vi "ADIS16470 Loop.vi"(8 "error in":errorcluster) -> ()   [LabVIEW 2019]
uses:
  Typedef/ADIS16470 Device Reference.ctl
  Typedef/ADIS16470 Hardware Configuration.ctl
  <vilib>/Rock Robotics/WPI/SPI/WPI_SPIMode.ctl
  <vilib>/Rock Robotics/SystemInterfaces/DIO/FPGA_DIOChannel.ctl
  <vilib>/Rock Robotics/SystemInterfaces/spilib/spi_bus.ctl
  Typedef/ADIS16470 Status.ctl
  Typedef/ADIS16470 Data.ctl
  Typedef/ADIS16470 Process.ctl
  Typedef/ADIS16470 Command Type.ctl
  <vilib>/Rock Robotics/SystemInterfaces/CounterEncoderSourceConvertion/FPGA_CounterEncoderSourceConvertionLVSourceType.ctl
  <vilib>/Rock Robotics/SystemInterfaces/DIO/FPGA_DIODigitalSourceChannel.ctl
  <vilib>/Rock Robotics/SystemInterfaces/AnalogTrigger/FPGA_AnalogTriggerIndex.ctl
  <vilib>/Rock Robotics/SystemInterfaces/AnalogTrigger/FPGA_AnalogTriggerOutType.ctl
  Typedef/ADIS16470 Calibration Time.ctl
  Typedef/ADIS16470 Loop Data.ctl
  <vilib>/Rock Robotics/WPI/SPI/WPI_SPIDevRef.ctl
  Typedef/ADIS16470 Register.ctl
  Typedef/ADIS16470 Loop State.ctl
  Typedef/ADIS16470 Register Read Info.ctl
  <vilib>/Rock Robotics/WPI/Counter/WPI_CounterDigitalInputToDigitalSource.vi
  <vilib>/Rock Robotics/WPI/ThirdParty/JAS_Junk/TrajLib/Trajectory_Library.lvlib
panel:
  in  "Use Register Read Mode":bool
  in  "Calibration Time":T1
  in  "element":T2
  out "Offset Bias":i16[](array[numeric])
  in  "ADIS16470DevRef":T3={"DevStatus"={"status"=FALSE, "code"=0, "source"=""}, "Hardware Config"={"SPI Clock Rate (Hz)"=1000000.0, "IMU SPI Mode (3)"=enum."Mode 3 (Clk Idle High,Sample on Trailing)", "IMU Reset Pin"=enum."SPI Port CS2", "IMU SPI Bus"=enum."SPI On-Board, CS0", "IMU Data Ready Pin"=enum."SPI Port CS1", "Stall Config"={"Pow2BytesPerRead"=255, "StallTicks"=640, "CsToSclkTicks"=5}}, "Calibration Complete"=refnum, "Status FIFO"=refnum, "Last Value Reference"=refnum, "Sychronous Process VI"=refnum, "Cmd FIFO"=refnum, "Source"={"DevStatus"={"status"=FALSE, "code"=0, "source"=""}, "AnalogTriggerMode?"=FALSE, "DigitalMode"={"DIO Channel"=enum."Disabled"}, "AnalogTriggerMode"={"AnalogTriggerIndex"=enum."Trig 0", "OutputType"=enum."InWindow"}}, "Data FIFO"=refnum, "Calibration Time"=enum."1s"}
  in  "Main Name":string
  # "XG_BIAS_LOW"
  # "XG_BIAS_HIGH"
  # "YG_BIAS_LOW"
  # "YG_BIAS_HIGH"
  # "ZG_BIAS_LOW"
  # "ZG_BIAS_HIGH"
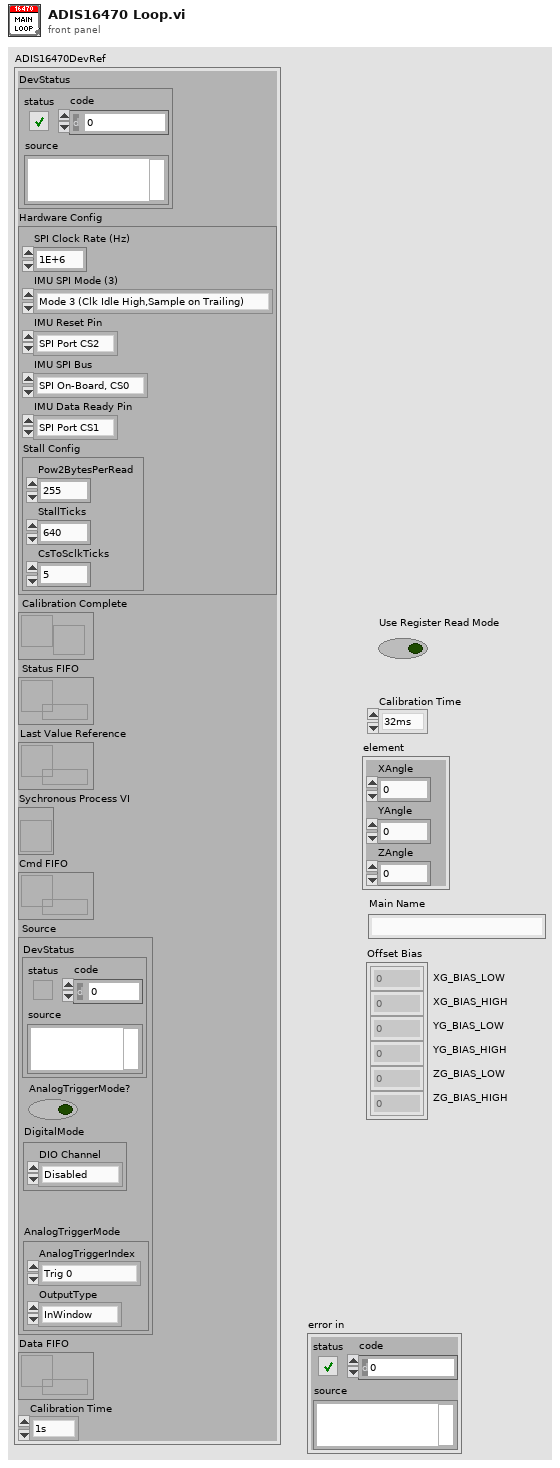
[diagram p1: front panel]
types:
  T1 = typedef "ADIS16470 Calibration Time.ctl" = enum16{"32ms", "64ms", "128ms", "256ms", "512ms", "1s", "2s", "4s", "8s", "16s", "32s", "64s"}
  T2 = typedef "ADIS16470 Data.ctl" = cluster{"XAngle":dbl, "YAngle":dbl, "ZAngle":dbl}
  T3 = typedef "ADIS16470 Device Reference.ctl" = cluster{"DevStatus":errorcluster, "Hardware Config":T4, "Calibration Complete":refnum<notifier>, "Status FIFO":refnum<k33>, "Last Value Reference":refnum<data-value>, "Sychronous Process VI":T8, "Cmd FIFO":refnum<k33>, "Source":T9, "Data FIFO":refnum<k33>, "Calibration Time":T1}
  T4 = typedef "ADIS16470 Hardware Configuration.ctl" = cluster{"SPI Clock Rate (Hz)":dbl, "IMU SPI Mode (3)":T5, "IMU Reset Pin":T6, "IMU SPI Bus":T7, "IMU Data Ready Pin":T6, "Stall Config":cluster{"Pow2BytesPerRead":u8, "StallTicks":u16, "CsToSclkTicks":u8}}
  T5 = typedef "WPI_SPIMode.ctl" = enum16{"Mode 0 (Clk Idle Low,Sample on Leading)", "Mode 1 (Clk Idle Low,Sample on Trailing)", "Mode 2 (Clk Idle High,Sample on Leading)", "Mode 3 (Clk Idle High,Sample on Trailing)"}
  T6 = typedef "FPGA_DIOChannel.ctl" = enum8{"DIO 0", "DIO 1", "DIO 2", "DIO 3", "DIO 4", "DIO 5", "DIO 6", "DIO 7", "DIO 8", "DIO 9", "DIO MXP 0", "DIO MXP 1", "DIO MXP 2", "DIO MXP 3", "DIO MXP 4", "DIO MXP 5", "DIO MXP 6", "DIO MXP 7", "DIO MXP 8", "DIO MXP 9", "DIO MXP 10", "DIO MXP 11", "DIO MXP 12", "DIO MXP 13", "DIO MXP 14", "DIO MXP 15", "SPI Port CS1", "SPI Port CS2", "SPI Port CS3", "SPI Port MISO", "SPI Port MOSI", "Invalid"}
  T7 = typedef "spi_bus.ctl" = enum16{"SPI On-Board, CS0", "SPI On-Board, CS1", "SPI On-Board, CS2", "SPI On-Board, CS3", "SPI MXP", "Invalid"}
  T8 = typedef "ADIS16470 Process.ctl" = refnum<vi>
  T9 = typedef "FPGA_CounterEncoderSourceConvertionLVSourceType.ctl" = cluster{"DevStatus":errorcluster, "AnalogTriggerMode?":bool, "DigitalMode":cluster{"DIO Channel":T10}, "AnalogTriggerMode":cluster{"AnalogTriggerIndex":T11, "OutputType":T12}}
  T10 = typedef "FPGA_DIODigitalSourceChannel.ctl" = enum8{"DIO 0", "DIO 1", "DIO 2", "DIO 3", "DIO 4", "DIO 5", "DIO 6", "DIO 7", "DIO 8", "DIO 9", "DIO MXP 0", "DIO MXP 1", "DIO MXP 2", "DIO MXP 3", "DIO MXP 4", "DIO MXP 5", "DIO MXP 6", "DIO MXP 7", "DIO MXP 8", "DIO MXP 9", "DIO MXP 10", "DIO MXP 11", "DIO MXP 12", "DIO MXP 13", "DIO MXP 14", "DIO MXP 15", "SPI Port CS1", "SPI Port CS2", "SPI Port CS3", "SPI Port MISO", "SPI Port MOSI", "Disabled"}
  T11 = typedef "FPGA_AnalogTriggerIndex.ctl" = enum8{"Trig 0", "Trig 1", "Trig 2", "Trig 3", "Trig 4", "Trig 5", "Trig 6", "Trig 7", "Invalid"}
  T12 = typedef "FPGA_AnalogTriggerOutType.ctl" = enum16{"InWindow", "TriggerState", "Rising", "Falling"}
  T13 = typedef "ADIS16470 Register Read Info.ctl" = cluster{"Reg":T14, "ByteInx":i32}[]
  T14 = typedef "ADIS16470 Register.ctl" = u8
  T15 = typedef "ADIS16470 Loop State.ctl" = enum16{"Default", "Error", "**Initialization**", "Reset", "Register DR Source", "Start SPI", "Write Config", "** Calibration **", "Calibrate", "Write Run Config", "Init Auto SPI", "** Operation **", "Run", "Process", "Run Cmds", "** Register Read Operation **", "Run Alt", "Run Cmds Alt"}
  T16 = typedef "ADIS16470 Loop Data.ctl" = cluster{"SPIDevRef":T17, "Data Counter":u16, "Reset":bool, "Digital Source":T9, "Bytes Per Sample":u32, "Data":dbl[], "ADIS16470DevRef":T3, "TimeStampPrev":u32, "Sensor to Robot Rotation":dbl[][], "Data Packet":T14[], "AutoSPI Active?":bool}
  T17 = typedef "WPI_SPIDevRef.ctl" = cluster{"DevStatus":errorcluster, "Handle":i32, "SPI Bus":T7}
  T18 = enum32{"Bad", "Idle", "Run top level", "Running"}
  T19 = typedef "ADIS16470 Status.ctl" = cluster{"Calibrated?":bool, "IMU Detected?":bool}
  T20 = typedef "ADIS16470 Command Type.ctl" = cluster{"Command":enum16{"None", "Reset", "Set Calibration Period", "Recalibrate", "Recal Complete", "Exit Auto SPI", "Start Auto SPI"}, "Data":u32}
  T21 = typedef "WPI_DigitalOutputDevRef.ctl" = cluster{"DIO Channel":T6, "DevStatus":errorcluster}
  T22 = typedef "WPI_DigitalInputDevRef.ctl" = cluster{"DevStatus":errorcluster, "DIO Channel":T6}
  T23 = cluster{"Pow2BytesPerRead":u8, "StallTicks":u16, "CsToSclkTicks":u8}
  T24 = enum16{"None", "Reset", "Set Calibration Period", "Recalibrate", "Recal Complete", "Exit Auto SPI", "Start Auto SPI"}
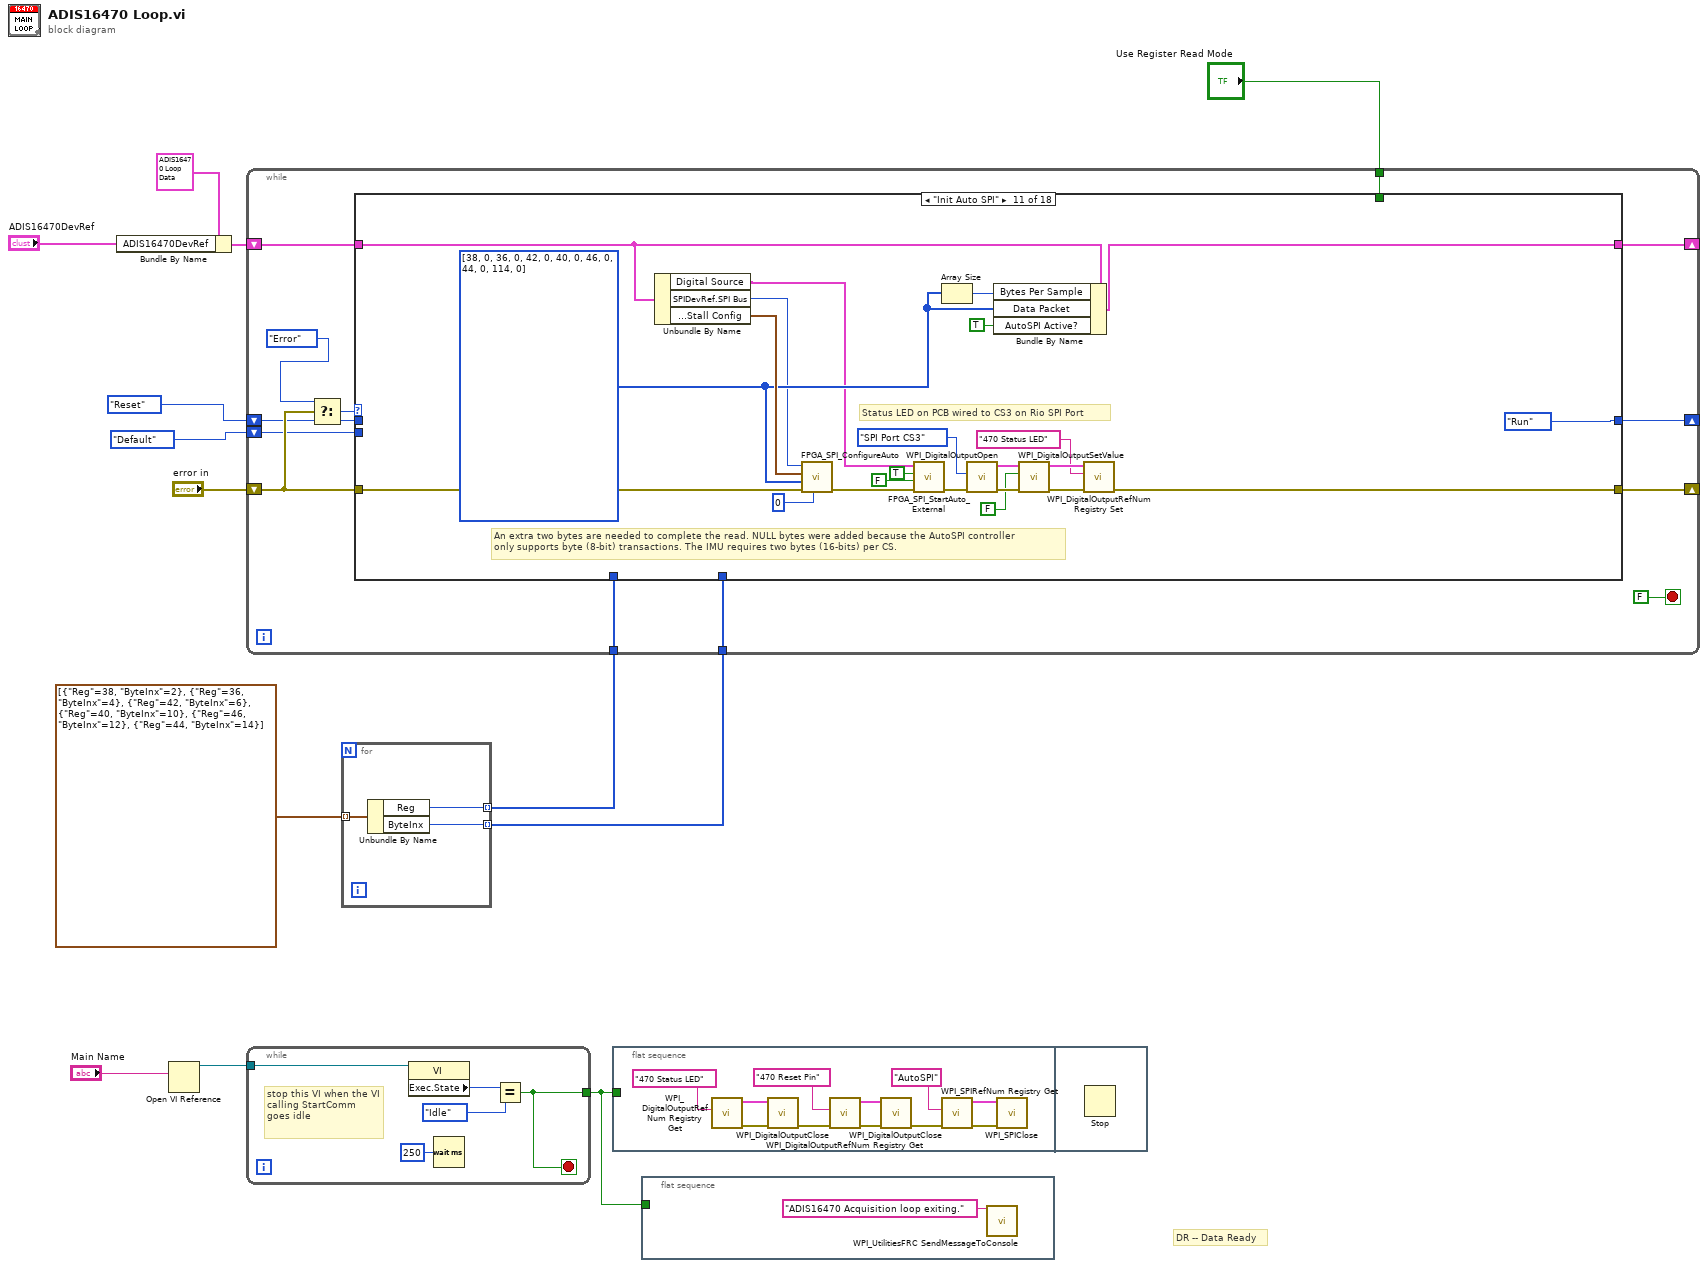
[diagram p0: block diagram]
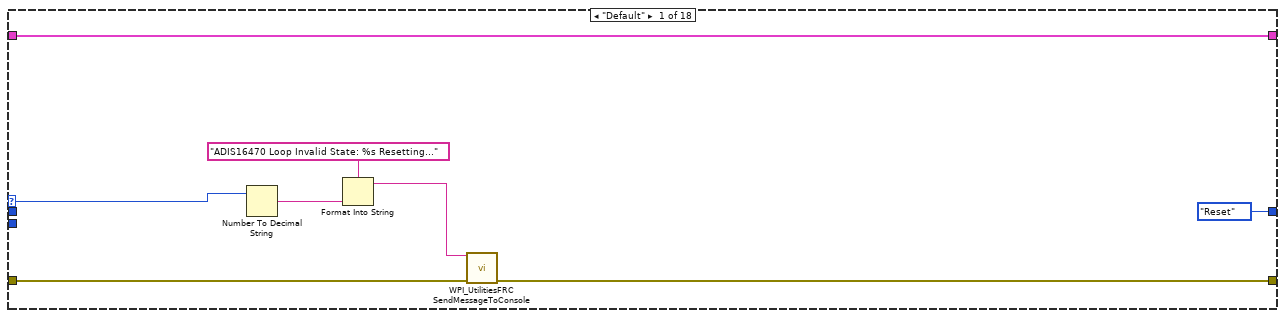
[diagram p2: hidden frame]
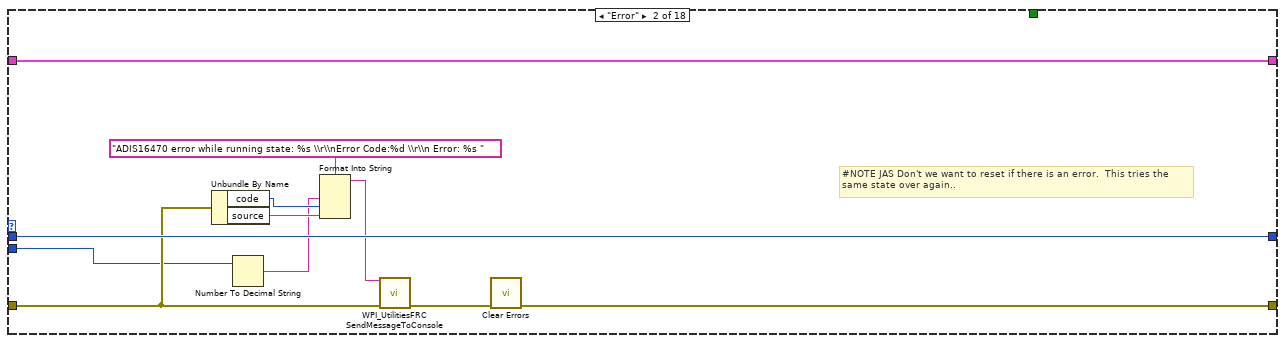
[diagram p3: hidden frame]
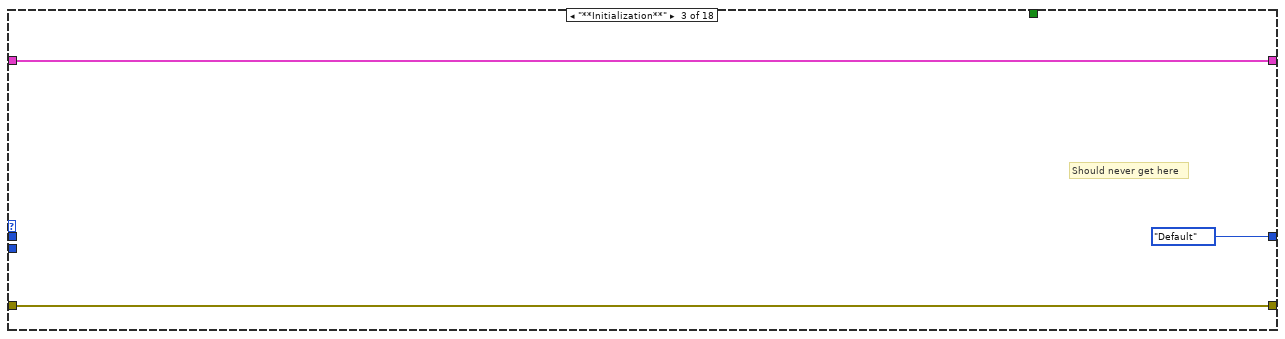
[diagram p4: hidden frame]
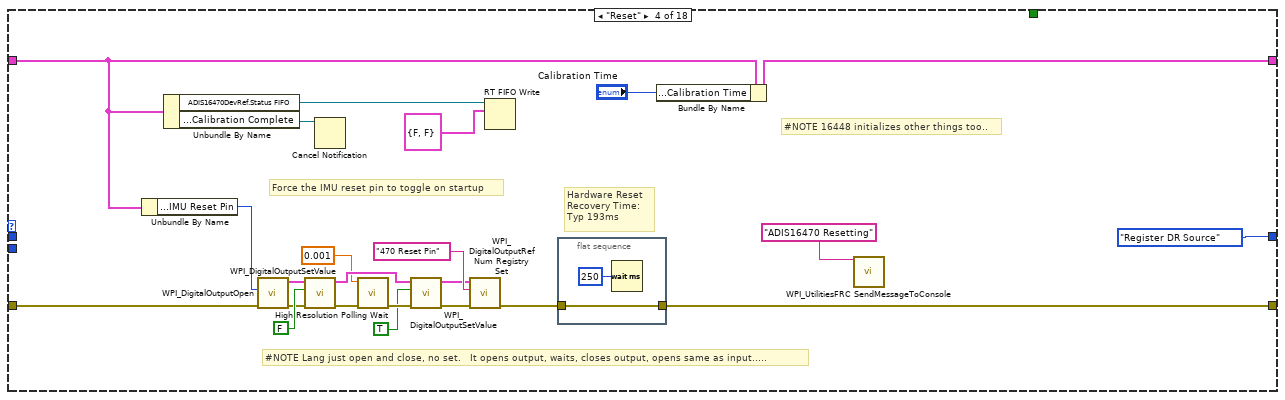
[diagram p5: hidden frame]
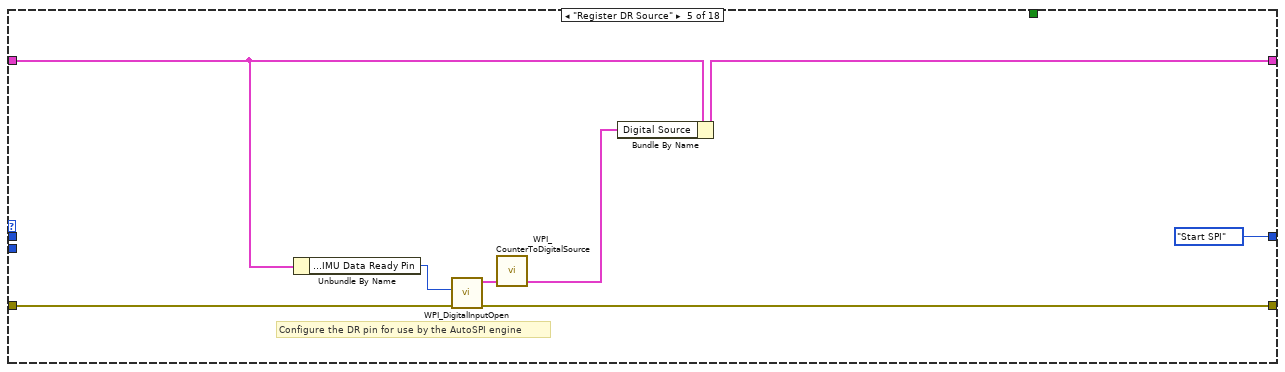
[diagram p6: hidden frame]
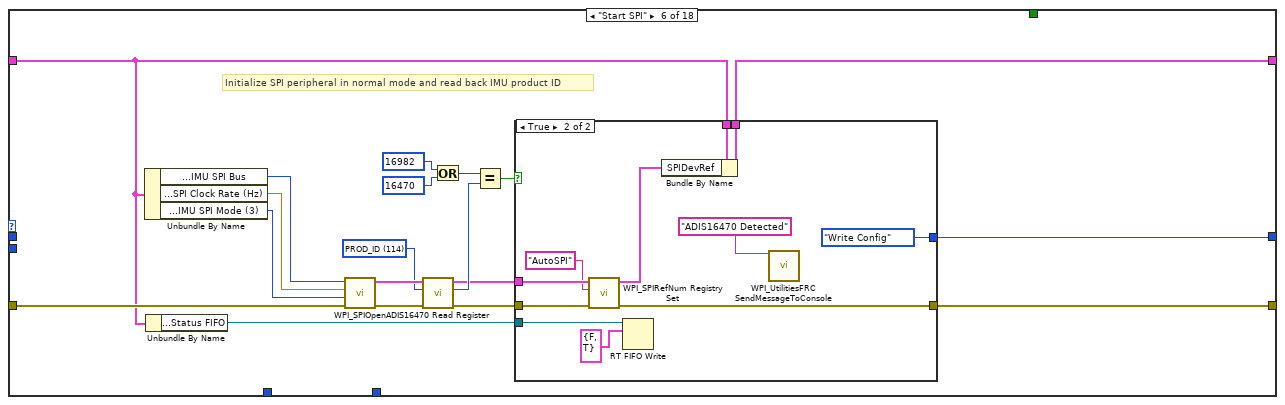
[diagram p7: hidden frame]
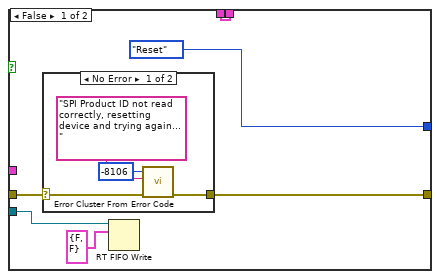
[diagram p8: hidden frame]
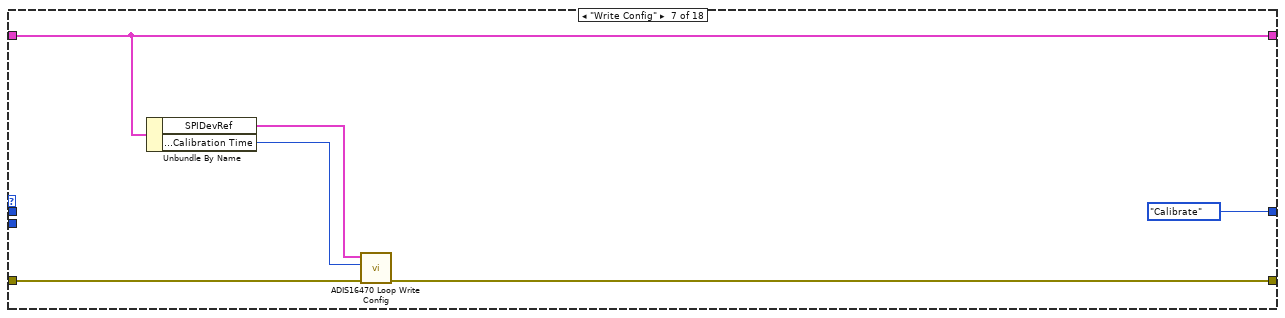
[diagram p10: hidden frame]
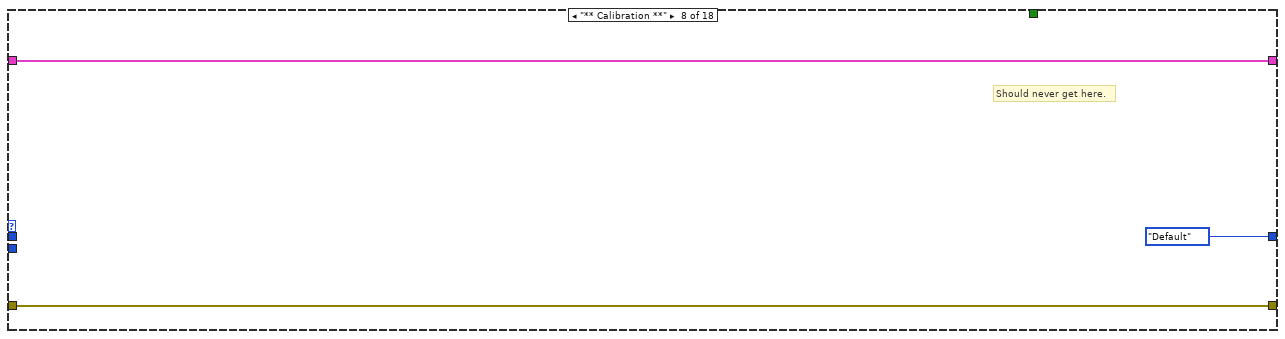
[diagram p11: hidden frame]
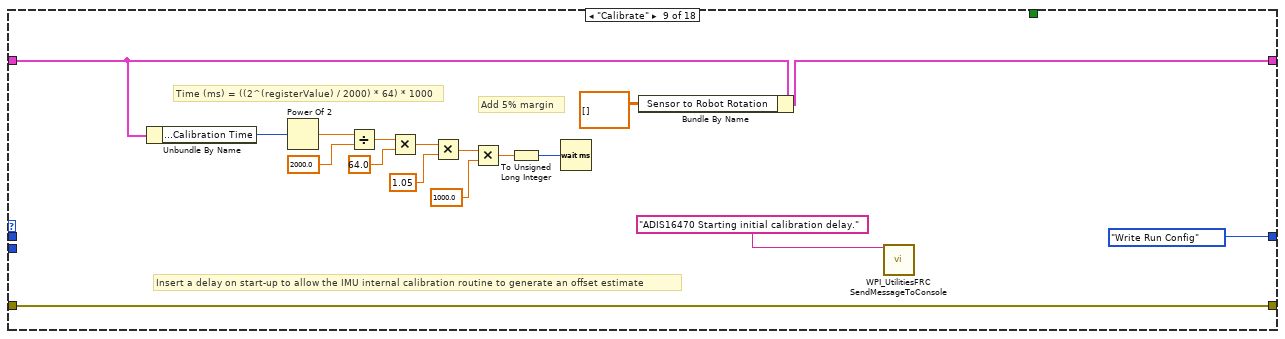
[diagram p12: hidden frame]
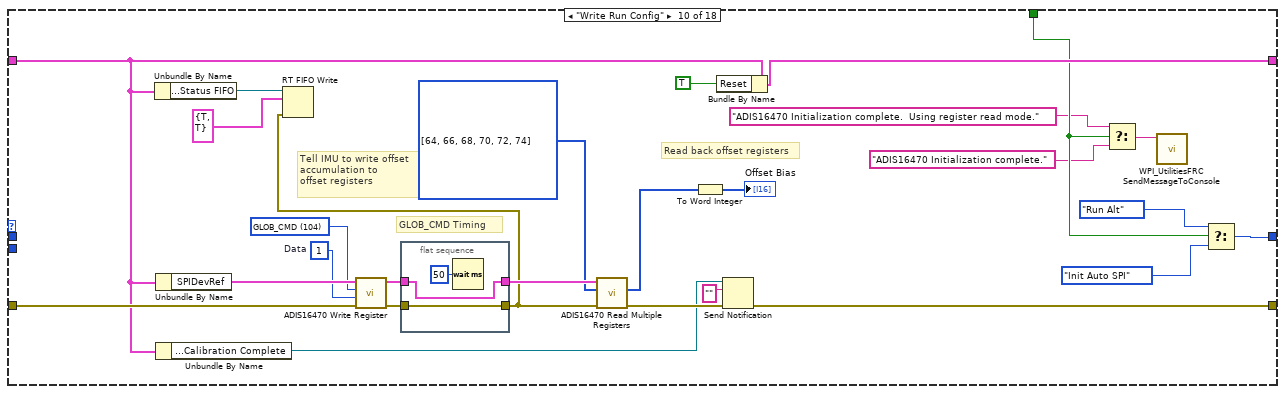
[diagram p13: hidden frame]
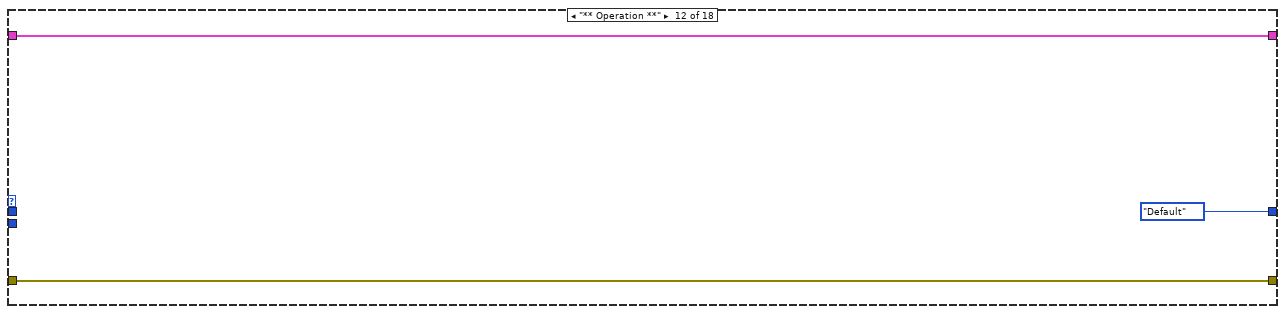
[diagram p14: hidden frame]
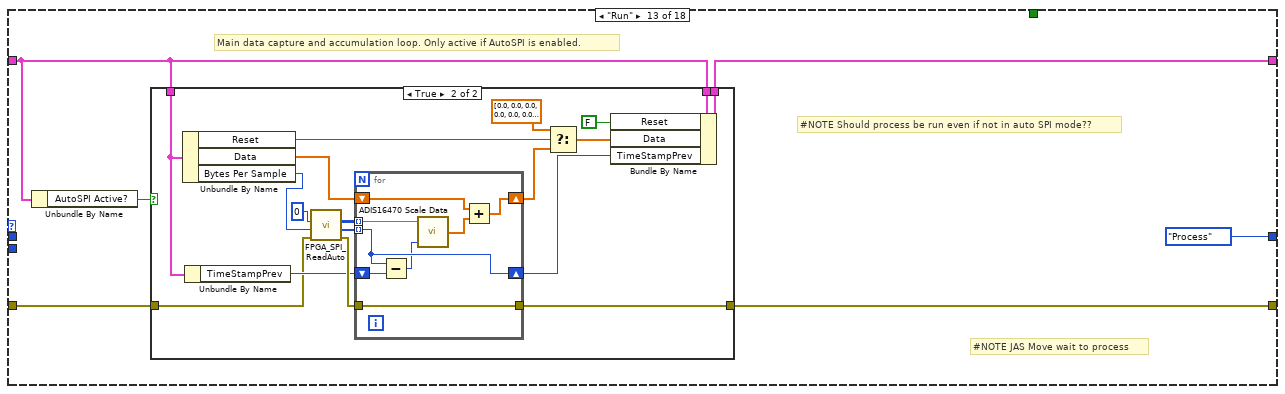
[diagram p15: hidden frame]
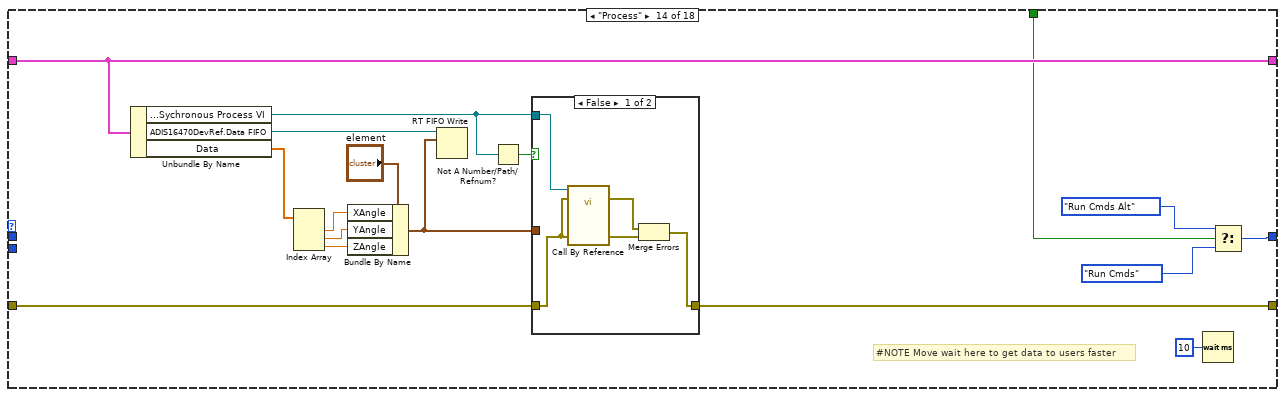
[diagram p17: hidden frame]
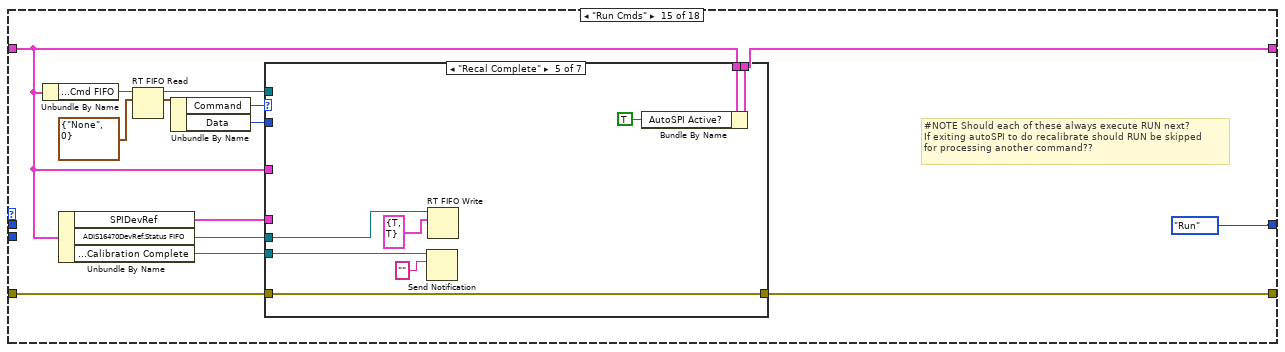
[diagram p19: hidden frame]
diagram:
  # "DR -- Data Ready"
  n1 = Bundle By Name(cluster=T16 {"SPIDevRef"={"DevStatus"={"status"=FALSE, "code"=0, "source"=""}, "Handle"=0, "SPI Bus"=enum."SPI On-Board, CS0"}, "Data Counter"=0, "Reset"=FALSE, "Digital Source"={"DevStatus"={"status"=FALSE, "code"=0, "source"=""}, "AnalogTriggerMode?"=FALSE, "DigitalMode"={"DIO Channel"=enum."DIO 1"}, "AnalogTriggerMode"={"AnalogTriggerIndex"=enum."Trig 0", "OutputType"=enum."InWindow"}}, "Bytes Per Sample"=0, "Data"=[0.0, 0.0, 0.0, 0.0, 0.0, 0.0, 0.0, 0.0], "ADIS16470DevRef"={"DevStatus"={"status"=FALSE, "code"=0, "source"=""}, "Hardware Config"={"SPI Clock Rate (Hz)"=1000000.0, "IMU SPI Mode (3)"=enum."Mode 3 (Clk Idle High,Sample on Trailing)", "IMU Reset Pin"=enum."SPI Port CS2", "IMU SPI Bus"=enum."SPI On-Board, CS0", "IMU Data Ready Pin"=enum."SPI Port CS1", "Stall Config"={"Pow2BytesPerRead"=255, "StallTicks"=640, "CsToSclkTicks"=5}}, "Calibration Complete"=refnum, "Status FIFO"=refnum, "Last Value Reference"=refnum, "Sychronous Process VI"=refnum, "Cmd FIFO"=refnum, "Source"={"DevStatus"={"status"=FALSE, "code"=0, "source"=""}, "AnalogTriggerMode?"=FALSE, "DigitalMode"={"DIO Channel"=enum."Disabled"}, "AnalogTriggerMode"={"AnalogTriggerIndex"=enum."Trig 0", "OutputType"=enum."InWindow"}}, "Data FIFO"=refnum, "Calibration Time"=enum."1s"}, "TimeStampPrev"=0, "Sensor to Robot Rotation"=[], "Data Packet"=[38, 0, 36, 0, 42, 0, 40, 0, 46, 0, 44, 0, 114, 0], "AutoSPI Active?"=TRUE}, "ADIS16470DevRef"="ADIS16470DevRef") -> (w10:T16)
  n2 = Open VI Reference(vi path="Main Name") -> (vi reference=w13:refnum<vi>)  [unwired: 3 in, 3 out]
  n3 = while {
    tunnel: w13 -> [w15]
    tunnel: [w14] -> w7
    stop <- w14 stop-if-true
    # "stop this VI when the VI calling StartComm goes idle"
    n4 = property class="VI"(reference=w15) -> ("Exec.State"=w17:T18)  [unwired: 1 in, 2 out]
    n5 = Wait (ms)(milliseconds to wait=u32 250) -> ()  [unwired: 1 out]
    n6 = Equal?(x=w17, y=T18."Idle" ("Execution:State")) -> (x = y?=w14:bool)
  }
  n7 = for {
    tunnel: T13 [{"Reg"=38, "ByteInx"=2}, {"Reg"=36, "ByteInx"=4}, {"Reg"=42, "ByteInx"=6}, {"Reg"=40, "ByteInx"=10}, {"Reg"=46, "ByteInx"=12}, {"Reg"=44, "ByteInx"=14}] ("RegistersToRead") -> [w21] mode=indexing
    tunnel: [w20] -> w2 mode=indexing
    tunnel: [w19] -> w1 mode=indexing
    n8 = Unbundle By Name(w21) -> ("Reg"=w20:T14, "ByteInx"=w19:i32)
  }
  n9 = while {
    shift-right: [w30] -> _
    shift-left: ADIS16470_Loop_State."Reset" ("ADIS16470 Loop State") -> [w27]
    shift-right: [w32] -> _
    shift-left: w10 -> [w33]
    shift-right: [w31] -> _
    shift-left: "error in" -> [w29]
    shift-left: ADIS16470_Loop_State."Default" ("ADIS16470 Loop State") -> [w26]
    tunnel: "Use Register Read Mode" -> [w24]
    tunnel: w2 -> [w23]
    tunnel: w1 -> [w22]
    stop <- FALSE stop-if-true
    n10 = Select(t=ADIS16470_Loop_State."Error" ("ADIS16470 Loop State"), s=w29, f=w27) -> (s? t:f=w28:T15)
    n11 = case shown="\"Init Auto SPI\"" w28 {
      selector: w28 -> [w36 _ _ _ _ _ _ _ _ _ _ _ _ _ _ _ _ _]
      tunnel: w33 -> [w42 w53 w56 w61 w86 w91 w134 w139 w153 w169 w202 w212 w215 w263 w272 w386 w406 w419]
      tunnel: [w42 w53 w56 w60 w89 w99 w134 w139 w155 w176 w201 w212 w218 w263 w279 w386 w409 w426] -> w32
      tunnel: w29 -> [w41 w49 w55 w77 w88 w105 w136 w138 w154 w182 w209 w211 w217 w261 w281 w385 w408 w428]
      tunnel: [w40 w50 w55 w76 w83 w98 w135 w138 w154 w171 w193 w211 w216 w260 w280 w385 w407 w427] -> w31
      tunnel: [ADIS16470_Loop_State."Reset" ("ADIS16470 Loop State") w52 ADIS16470_Loop_State."Default" ("ADIS16470 Loop State") ADIS16470_Loop_State."Register DR Source" ("ADIS16470 Loop State") ADIS16470_Loop_State."Start SPI" ("ADIS16470 Loop State") w100 ADIS16470_Loop_State."Calibrate" ("ADIS16470 Loop State") ADIS16470_Loop_State."Default" ("ADIS16470 Loop State") ADIS16470_Loop_State."Write Run Config" ("ADIS16470 Loop State") w162 ADIS16470_Loop_State."Run" ("ADIS16470 Loop State") ADIS16470_Loop_State."Default" ("ADIS16470 Loop State") ADIS16470_Loop_State."Process" ("ADIS16470 Loop State") w250 ADIS16470_Loop_State."Run" ("ADIS16470 Loop State") ADIS16470_Loop_State."Default" ("ADIS16470 Loop State") ADIS16470_Loop_State."Process" ("ADIS16470 Loop State") ADIS16470_Loop_State."Run Alt" ("ADIS16470 Loop State")] -> w30
      tunnel: w27 -> [_ w52 _ _ _ _ _ _ _ _ _ _ _ _ _ _ _ _]
      tunnel: w26 -> [_ w44 _ _ _ _ _ _ _ _ _ _ _ _ _ _ _ _]
      tunnel: w24 -> [_ _ _ _ _ _ _ _ _ w160 _ _ _ w247 _ _ _ _]
      tunnel: w23 -> [_ _ _ _ _ _ _ _ _ _ _ _ _ _ _ _ w404 _]
      tunnel: w22 -> [_ _ _ _ _ _ _ _ _ _ _ _ _ _ _ _ w390 _]
      frame "Default" {
        n12 = Number To Decimal String(number=w36) -> (decimal integer string=w35:string)  [unwired: 1 in]
        n13 = Format Into String(format string="ADIS16470 Loop Invalid State: %s Resetting...", w35) -> (resulting string=w39:string)  [unwired: 2 in, 1 out]
        n14 = call <vilib>:"WPI_UtilitiesFRC SendMessageToConsole.vi"("Message"=w39, "error in (no error)"=w41) -> ("error out"=w40:errorcluster)  [unwired: 13 in]
      }
      frame "Error" {
        # "#NOTE JAS Don't we want to reset if there is an error.  This tries the\nsame state over again.."
        n15 = Unbundle By Name(w49) -> ("code"=w46:i32, "source"=w45:string)
        n16 = Number To Decimal String(number=w44) -> (decimal integer string=w43:string)  [unwired: 1 in]
        n17 = Format Into String(format string="ADIS16470 error while running state: %s \\r\\nError Code:%d \\r\\n Error: %s ", w43, w46, w45) -> (resulting string=w48:string)  [unwired: 2 in, 1 out]
        n18 = call <vilib>:"WPI_UtilitiesFRC SendMessageToConsole.vi"("Message"=w48, "error in (no error)"=w49) -> ("error out"=w51:errorcluster)  [unwired: 13 in]
        n19 = call <vilib>:"Clear Errors.vi"("error in (no error)"=w51) -> ("error out"=w50:errorcluster)  [unwired: 5 in, 1 out]
      }
      frame "**Initialization**" {
        # "Should never get here"
      }
      frame "Reset" {
        # "#NOTE Lang just open and close, no set.   It opens output, waits, closes output, opens same as input....."
        # "#NOTE 16448 initializes other things too.."
        # "Hardware Reset Recovery Time: Typ 193ms"
        # "Force the IMU reset pin to toggle on startup"
        n20 = Unbundle By Name(w61) -> ("ADIS16470DevRef.Hardware Config.IMU Reset Pin"=w78:T6)
        n21 = Unbundle By Name(w61) -> ("ADIS16470DevRef.Status FIFO"=w74:refnum<k33>, "ADIS16470DevRef.Calibration Complete"=w75:refnum<notifier>)
        n22 = call <vilib>:"WPI_DigitalOutputOpen.vi"("error in (no error)"=w77, "DIO Channel"=w78) -> ("error out"=w71:errorcluster, "DigitalOutputDevRef"=w79:T21)  [unwired: 8 in]
        n23 = call <vilib>:"WPI_DigitalOutputSetValue.vi"("error in (no error)"=w71, "Value"=FALSE, "DigitalOutputDevRef"=w79) -> ("error out"=w68:errorcluster, "DigitalOutputDevRef"=w66:T21)  [unwired: 7 in]
        n24 = Cancel Notification(0:w75) -> ()  [unwired: 1 in, 3 out]
        n25 = call <vilib>:"High Resolution Polling Wait.vi"("error in (no error)"=w68, "seconds to wait"=0.001) -> ("error out"=w67:errorcluster)  [unwired: 9 in]
        n26 = call <vilib>:"WPI_DigitalOutputSetValue.vi"("error in (no error)"=w67, "Value"=TRUE, "DigitalOutputDevRef"=w66) -> ("error out"=w63:errorcluster, "DigitalOutputDevRef"=w64:T21)  [unwired: 7 in]
        n27 = call <vilib>:"WPI_DigitalOutputRefNum Registry Set.vi"("error in (no error)"=w63, "refnum name"="470 Reset Pin", "DigitalOutputDevRef"=w64) -> ("error out"=w69:errorcluster)  [unwired: 7 in, 1 out]
        n28 = RT FIFO Write(0:w74, 1:T19 {"Calibrated?"=FALSE, "IMU Detected?"=FALSE} ("element")) -> ()  [unwired: 3 in, 4 out]
        n29 = flat-sequence {
          tunnel: [w81] -> w76
          tunnel: w69 -> [w81]
          frame #0 {
            n30 = Wait (ms)(milliseconds to wait=u32 250) -> ()  [unwired: 1 out]
          }
        }
        n31 = Bundle By Name(cluster=w61, "ADIS16470DevRef.Calibration Time"="Calibration Time") -> (w60:T16)
        n32 = call <vilib>:"WPI_UtilitiesFRC SendMessageToConsole.vi"("Message"="ADIS16470 Resetting" ("format string")) -> ()  [unwired: 14 in, 1 out]
      }
      frame "Register DR Source" {
        # "Configure the DR pin for use by the AutoSPI engine"
        n33 = Unbundle By Name(w86) -> ("ADIS16470DevRef.Hardware Config.IMU Data Ready Pin"=w85:T6)
        n34 = call <vilib>:"WPI_DigitalInputOpen.vi"("error in (no error)"=w88, "DIO Channel"=w85) -> ("error out"=w83:errorcluster, "DigitalInputDevRef"=w87:T22)  [unwired: 8 in]
        n35 = call-poly <vilib>:"WPI_CounterToDigitalSource.vi"("DigitalInputDevRef"=w87) -> ("Digital Source"=w84:T9)  [unwired: 6 in]
        n36 = Bundle By Name(cluster=w86, "Digital Source"=w84) -> (w89:T16)
      }
      frame "Start SPI" {
        w93 = T14 114 items=["Reserved1"=0, "DIAG_STAT"=2, "X_GYRO_LOW"=4, "X_GYRO_OUT"=6, "Y_GYRO_LOW"=8, "Y_GYRO_OUT"=10, "Z_GYRO_LOW"=12, "Z_GYRO_OUT"=14, "X_ACCL_LOW"=16, "X_ACCL_OUT"=18, "Y_ACCL_LOW"=20, "Y_ACCL_OUT"=22, "Z_ACCL_LOW"=24, "Z_ACCL_OUT"=26, "TEMP_OUT"=28, "TIME_STAMP"=30, "Reseved2"=32, "DATA_CNTR"=34, "X_DELTANG_LOW"=36, "X_DELTANG_OUT"=38, "Y_DELTANG_LOW"=40, "Y_DELTANG_OUT"=42, "Z_DELTANG_LOW"=44, "Z_DELTANG_OUT"=46, "X_DELTVEL_LOW"=48, "X_DELTVEL_OUT"=50, "Y_DELTVEL_LOW"=52, "Y_DELTVEL_OUT"=54, "Z_DELTVEL_LOW"=56, "Z_DELTVEL_OUT"=58, "Reserved3"=60, "Reserved4"=62, "XG_BIAS_LOW"=64, "XG_BIAS_HIGH"=66, "YG_BIAS_LOW"=68, "YG_BIAS_OUT"=70, "ZG_BIAS_LOW"=72, "ZG_BIAS_OUT"=74, "XA_BIAS_LOW"=76, "XA_BIAS_HIGH"=78, "YA_BIAS_LOW"=80, "YA_BIAS_OUT"=82, "ZA_BIAS_LOW"=84, "ZA_BIAS_OUT"=86, "Reserved5"=88, "Reserved6"=90, "FILT_CTRL"=92, "Reserved5"=94, "MSC_CTRL"=96, "UP_SCALE"=98, "DEC_RATE"=100, "NULL_CNFG"=102, "GLOB_CMD"=104, "Reserved6"=106, "FIRM_REV"=108, "FIRM_DM"=110, "FIRM_Y"=112, "PROD_ID"=114, "SERIAL_NUM"=116, "USER_SCR1"=118, "USER_SCR2"=120, "USER_SCR3"=122, "FLSHCNT_LOW"=124, "FLSHCNT_HIGH"=126] ("ADIS16448 Register")
        # "Initialize SPI peripheral in normal mode and read back IMU product ID"
        n37 = Unbundle By Name(w91) -> ("ADIS16470DevRef.Hardware Config.IMU SPI Bus"=w101:T7, "ADIS16470DevRef.Hardware Config.SPI Clock Rate (Hz)"=w102:dbl, "ADIS16470DevRef.Hardware Config.IMU SPI Mode (3)"=w103:T5)
        n38 = Unbundle By Name(w91) -> ("ADIS16470DevRef.Status FIFO"=w90:refnum<k33>)
        n39 = call <vilib>:"WPI_SPIOpen.vi"("error in"=w105, "Mode (3)"=w103, "Clock Rate (Hz)"=w102, "SPI Bus"=w101) -> ("error out"=w95:errorcluster, "SPIDevRef"=w94:T17)  [unwired: 6 in]
        n40 = call "ADIS16470 Read Register.vi"("error in (no error)"=w95, "ADIS16470 Register"=w93, "SPIDevRef in"=w94) -> ("error out"=w96:errorcluster, "Register Value"=w97:u16, "SPIDevRef out"=w92:T17)  [unwired: 6 in]
        n41 = Or(x=u16 16982 ("y"), y=u16 16470) -> (x .or. y?=w106:u16)
        n42 = Equal?(x=w106, y=w97) -> (x = y?=w104:bool)
        n43 = case shown="True" w104 {
          tunnel: [ADIS16470_Loop_State."Reset" ("ADIS16470 Loop State") ADIS16470_Loop_State."Write Config" ("ADIS16470 Loop State")] -> w100
          tunnel: w91 -> [w114 w130]
          tunnel: [w114 w129] -> w99
          tunnel: [w113 w125] -> w98
          tunnel: w96 -> [w112 w128]
          tunnel: w92 -> [_ w127]
          tunnel: w90 -> [w110 w123]
          frame False {
            n44 = case shown="No Error" w112 {
              selector: w112 -> [w117 w119]
              tunnel: [w118 w119] -> w113
              frame No Error {
                n45 = call <vilib>:"Error Cluster From Error Code.vi"("error in (no error)"=w117, "error message (\"\")"="SPI Product ID not read correctly, resetting device and trying again..." ("error message (\"\")"), "error code (0)"=-8106) -> ("error out"=w118:errorcluster)  [unwired: 6 in]
              }
              frame Error {
              }
            }
            n46 = RT FIFO Write(0:w110, 1:T19 {"Calibrated?"=FALSE, "IMU Detected?"=FALSE} ("element")) -> ()  [unwired: 3 in, 4 out]
          }
          frame True {
            n47 = call <vilib>:"WPI_SPIRefNum Registry Set.vi"("error in (no error)"=w128, "refnum name"="AutoSPI", "SPIDevRef"=w127) -> ("error out"=w125:errorcluster, "SPIDevRef"=w126:T17)  [unwired: 7 in]
            n48 = RT FIFO Write(0:w123, 1:T19 {"Calibrated?"=FALSE, "IMU Detected?"=TRUE} ("element")) -> ()  [unwired: 3 in, 4 out]
            n49 = Bundle By Name(cluster=w130, "SPIDevRef"=w126) -> (w129:T16)
            n50 = call <vilib>:"WPI_UtilitiesFRC SendMessageToConsole.vi"("Message"="ADIS16470 Detected" ("format string")) -> ()  [unwired: 14 in, 1 out]
          }
        }
      }
      frame "Write Config" {
        n51 = Unbundle By Name(w134) -> ("SPIDevRef"=w132:T17, "ADIS16470DevRef.Calibration Time"=w131:T1)
        n52 = call "ADIS16470 Loop Write Config.vi"("error in (no error)"=w136, "Calibration Time"=w131, "SPIDevRef"=w132) -> ("error out"=w135:errorcluster)  [unwired: 8 in]
      }
      frame "** Calibration **" {
        # "Should never get here."
      }
      frame "Calibrate" {
        # "Insert a delay on start-up to allow the IMU internal calibration routine to generate an offset estimate"
        # "Add 5% margin"
        # "Time (ms) = ((2^(registerValue) / 2000) * 64) * 1000"
        n53 = Unbundle By Name(w153) -> ("ADIS16470DevRef.Calibration Time"=w152:T1)
        n54 = Power Of 2(x=w152) -> (2^x=w151:dbl)
        n55 = Divide(x=w151, y=2000.0) -> (x/y=w149:dbl)
        n56 = Multiply(x=w149, y=64.0) -> (x*y=w147:dbl)
        n57 = Multiply(x=w147, y=1.05) -> (x*y=w145:dbl)
        n58 = Multiply(x=w145, y=1000.0) -> (x*y=w141:dbl)
        n59 = To Unsigned Long Integer(number=w141) -> (unsigned 32bit integer=w140:u32)
        n60 = Wait (ms)(milliseconds to wait=w140) -> ()  [unwired: 1 out]
        n61 = Bundle By Name(cluster=w153, "Sensor to Robot Rotation"=dbl[][] []) -> (w155:T16)
        n62 = call <vilib>:"WPI_UtilitiesFRC SendMessageToConsole.vi"("Message"="ADIS16470 Starting initial calibration delay.") -> ()  [unwired: 14 in, 1 out]
      }
      frame "Write Run Config" {
        w166 = T14 104 items=["Reserved1"=0, "DIAG_STAT"=2, "X_GYRO_LOW"=4, "X_GYRO_OUT"=6, "Y_GYRO_LOW"=8, "Y_GYRO_OUT"=10, "Z_GYRO_LOW"=12, "Z_GYRO_OUT"=14, "X_ACCL_LOW"=16, "X_ACCL_OUT"=18, "Y_ACCL_LOW"=20, "Y_ACCL_OUT"=22, "Z_ACCL_LOW"=24, "Z_ACCL_OUT"=26, "TEMP_OUT"=28, "TIME_STAMP"=30, "Reseved2"=32, "DATA_CNTR"=34, "X_DELTANG_LOW"=36, "X_DELTANG_OUT"=38, "Y_DELTANG_LOW"=40, "Y_DELTANG_OUT"=42, "Z_DELTANG_LOW"=44, "Z_DELTANG_OUT"=46, "X_DELTVEL_LOW"=48, "X_DELTVEL_OUT"=50, "Y_DELTVEL_LOW"=52, "Y_DELTVEL_OUT"=54, "Z_DELTVEL_LOW"=56, "Z_DELTVEL_OUT"=58, "Reserved3"=60, "Reserved4"=62, "XG_BIAS_LOW"=64, "XG_BIAS_HIGH"=66, "YG_BIAS_LOW"=68, "YG_BIAS_OUT"=70, "ZG_BIAS_LOW"=72, "ZG_BIAS_OUT"=74, "XA_BIAS_LOW"=76, "XA_BIAS_HIGH"=78, "YA_BIAS_LOW"=80, "YA_BIAS_OUT"=82, "ZA_BIAS_LOW"=84, "ZA_BIAS_OUT"=86, "Reserved5"=88, "Reserved6"=90, "FILT_CTRL"=92, "Reserved5"=94, "MSC_CTRL"=96, "UP_SCALE"=98, "DEC_RATE"=100, "NULL_CNFG"=102, "GLOB_CMD"=104, "Reserved6"=106, "FIRM_REV"=108, "FIRM_DM"=110, "FIRM_Y"=112, "PROD_ID"=114, "SERIAL_NUM"=116, "USER_SCR1"=118, "USER_SCR2"=120, "USER_SCR3"=122, "FLSHCNT_LOW"=124, "FLSHCNT_HIGH"=126] ("Register")
        w181 = u16 1  # Data
        w177 = T14[] [64, 66, 68, 70, 72, 74] items=["Reserved1"=0, "DIAG_STAT"=2, "X_GYRO_LOW"=4, "X_GYRO_OUT"=6, "Y_GYRO_LOW"=8, "Y_GYRO_OUT"=10, "Z_GYRO_LOW"=12, "Z_GYRO_OUT"=14, "X_ACCL_LOW"=16, "X_ACCL_OUT"=18, "Y_ACCL_LOW"=20, "Y_ACCL_OUT"=22, "Z_ACCL_LOW"=24, "Z_ACCL_OUT"=26, "TEMP_OUT"=28, "TIME_STAMP"=30, "Reseved2"=32, "DATA_CNTR"=34, "X_DELTANG_LOW"=36, "X_DELTANG_OUT"=38, "Y_DELTANG_LOW"=40, "Y_DELTANG_OUT"=42, "Z_DELTANG_LOW"=44, "Z_DELTANG_OUT"=46, "X_DELTVEL_LOW"=48, "X_DELTVEL_OUT"=50, "Y_DELTVEL_LOW"=52, "Y_DELTVEL_OUT"=54, "Z_DELTVEL_LOW"=56, "Z_DELTVEL_OUT"=58, "Reserved3"=60, "Reserved4"=62, "XG_BIAS_LOW"=64, "XG_BIAS_HIGH"=66, "YG_BIAS_LOW"=68, "YG_BIAS_HIGH"=70, "ZG_BIAS_LOW"=72, "ZG_BIAS_HIGH"=74, "XA_BIAS_LOW"=76, "XA_BIAS_HIGH"=78, "YA_BIAS_LOW"=80, "YA_BIAS_HIGH"=82, "ZA_BIAS_LOW"=84, "ZA_BIAS_HIGH"=86, "Reserved5"=88, "Reserved6"=90, "FILT_CTRL"=92, "Reserved5"=94, "MSC_CTRL"=96, "UP_SCALE"=98, "DEC_RATE"=100, "NULL_CNFG"=102, "GLOB_CMD"=104, "Reserved6"=106, "FIRM_REV"=108, "FIRM_DM"=110, "FIRM_Y"=112, "PROD_ID"=114, "SERIAL_NUM"=116, "USER_SCR1"=118, "USER_SCR2"=120, "USER_SCR3"=122, "FLSHCNT_LOW"=124, "FLSHCNT_HIGH"=126] ("Registers")
        # "Tell IMU to write offset \naccumulation to \noffset registers"
        # "GLOB_CMD Timing"
        # "Read back offset registers"
        n63 = Unbundle By Name(w169) -> ("ADIS16470DevRef.Status FIFO"=w168:refnum<k33>)
        n64 = Unbundle By Name(w169) -> ("SPIDevRef"=w183:T17)
        n65 = Unbundle By Name(w169) -> ("ADIS16470DevRef.Calibration Complete"=w172:refnum<notifier>)
        n66 = RT FIFO Write(0:w168, 1:T19 {"Calibrated?"=TRUE, "IMU Detected?"=TRUE} ("element"), 3:w165) -> ()  [unwired: 2 in, 4 out]
        n67 = call "ADIS16470 Write Register.vi"("error in (no error)"=w182, "Data"=w181, "Register"=w166, "SPIDevRef in"=w183) -> ("error out"=w180:errorcluster, "SPIDevRef out"=w179:T17)  [unwired: 6 in]
        n68 = flat-sequence {
          tunnel: w180 -> [w186]
          tunnel: [w186] -> w165
          tunnel: w179 -> [w184]
          tunnel: [w184] -> w178
          frame #0 {
            n69 = Wait (ms)(milliseconds to wait=u32 50) -> ()  [unwired: 1 out]
          }
        }
        n70 = call "ADIS16470 Read Multiple Registers.vi"("error in (no error)"=w165, "Registers"=w177, "SPIDevRefIn"=w178) -> ("error out"=w173:errorcluster, "Values"=w164:u16[])  [unwired: 6 in, 1 out]
        n71 = To Word Integer(number=w164) -> (16bit integer=→"Offset Bias":i16[])
        n72 = Bundle By Name(cluster=w169, "Reset"=TRUE ("First Run")) -> (w176:T16)
        n73 = Send Notification(notification="", notifier=w172, error in (no error)=w173) -> (error out=w171:errorcluster)  [unwired: 1 out]
        n74 = Select(t="ADIS16470 Initialization complete.  Using register read mode." ("format string"), s=w160, f="ADIS16470 Initialization complete." ("format string")) -> (s? t:f=w157:string)
        n75 = call <vilib>:"WPI_UtilitiesFRC SendMessageToConsole.vi"("Message"=w157) -> ()  [unwired: 14 in, 1 out]
        n76 = Select(t=ADIS16470_Loop_State."Run Alt", s=w160, f=ADIS16470_Loop_State."Init Auto SPI" ("ADIS16470 Loop State")) -> (s? t:f=w162:T15)
      }
      frame "Init Auto SPI" {
        w190 = T14[] [38, 0, 36, 0, 42, 0, 40, 0, 46, 0, 44, 0, 114, 0] items=["NULL"=0, "DIAG_STAT"=2, "X_GYRO_LOW"=4, "X_GYRO_OUT"=6, "Y_GYRO_LOW"=8, "Y_GYRO_OUT"=10, "Z_GYRO_LOW"=12, "Z_GYRO_OUT"=14, "X_ACCL_LOW"=16, "X_ACCL_OUT"=18, "Y_ACCL_LOW"=20, "Y_ACCL_OUT"=22, "Z_ACCL_LOW"=24, "Z_ACCL_OUT"=26, "TEMP_OUT"=28, "TIME_STAMP"=30, "Reseved2"=32, "DATA_CNTR"=34, "X_DELTANG_LOW"=36, "X_DELTANG_OUT"=38, "Y_DELTANG_LOW"=40, "Y_DELTANG_OUT"=42, "Z_DELTANG_LOW"=44, "Z_DELTANG_OUT"=46, "X_DELTVEL_LOW"=48, "X_DELTVEL_OUT"=50, "Y_DELTVEL_LOW"=52, "Y_DELTVEL_OUT"=54, "Z_DELTVEL_LOW"=56, "Z_DELTVEL_OUT"=58, "Reserved3"=60, "Reserved4"=62, "XG_BIAS_LOW"=64, "XG_BIAS_HIGH"=66, "YG_BIAS_LOW"=68, "YG_BIAS_HIGH"=70, "ZG_BIAS_LOW"=72, "ZG_BIAS_HIGH"=74, "XA_BIAS_LOW"=76, "XA_BIAS_HIGH"=78, "YA_BIAS_LOW"=80, "YA_BIAS_HIGH"=82, "ZA_BIAS_LOW"=84, "ZA_BIAS_HIGH"=86, "Reserved5"=88, "Reserved6"=90, "FILT_CTRL"=92, "Reserved5"=94, "MSC_CTRL"=96, "UP_SCALE"=98, "DEC_RATE"=100, "NULL_CNFG"=102, "GLOB_CMD"=104, "Reserved6"=106, "FIRM_REV"=108, "FIRM_DM"=110, "FIRM_Y"=112, "PROD_ID"=114, "SERIAL_NUM"=116, "USER_SCR1"=118, "USER_SCR2"=120, "USER_SCR3"=122, "FLSHCNT_LOW"=124, "FLSHCNT_HIGH"=126] ("Registers")
        # "Status LED on PCB wired to CS3 on Rio SPI Port"
        # "An extra two bytes are needed to complete the read. NULL bytes were added because the AutoSPI controller \nonly supports byte (8-bit) transactions. The IMU requires two bytes (16-bits) per CS."
        n77 = Unbundle By Name(w202) -> ("Digital Source"=w189:T9, "SPIDevRef.SPI Bus"=w188:T7, "ADIS16470DevRef.Hardware Config.Stall Config"=w192:T23)
        n78 = call <vilib>:"FPGA_SPI_ConfigureAuto.vi"("SPI Auto Zero Byte Count"=u8 0, "error in"=w209, "SPI Auto TX Byte Array"=w190, "Stall Config"=w192, "SPI Bus"=w188) -> ("error out"=w207:errorcluster)  [unwired: 6 in]
        n79 = call <vilib>:"FPGA_SPI_StartAuto_External.vi"("error in (no error)"=w207, "Falling Edge"=FALSE, "Rising Edge"=TRUE, "Source"=w189) -> ("error out"=w203:errorcluster)  [unwired: 7 in]
        n80 = Array Size(array=w190) -> (size(s)=w200:i32)
        n81 = call <vilib>:"WPI_DigitalOutputOpen.vi"("error in (no error)"=w203, "DIO Channel"=FPGA_DIOChannel."SPI Port CS3") -> ("error out"=w199:errorcluster, "DigitalOutputDevRef"=w198:T21)  [unwired: 8 in]
        n82 = Bundle By Name(cluster=w202, "Bytes Per Sample"=w200, "Data Packet"=w190, "AutoSPI Active?"=TRUE) -> (w201:T16)
        n83 = call <vilib>:"WPI_DigitalOutputSetValue.vi"("error in (no error)"=w199, "Value"=FALSE, "DigitalOutputDevRef"=w198) -> ("error out"=w196:errorcluster, "DigitalOutputDevRef"=w195:T21)  [unwired: 7 in]
        n84 = call <vilib>:"WPI_DigitalOutputRefNum Registry Set.vi"("error in (no error)"=w196, "refnum name"="470 Status LED", "DigitalOutputDevRef"=w195) -> ("error out"=w193:errorcluster)  [unwired: 7 in, 1 out]
      }
      frame "** Operation **" {
      }
      frame "Run" {
        # "#NOTE Should process be run even if not in auto SPI mode??"
        # "#NOTE JAS Move wait to process"
        # "Main data capture and accumulation loop. Only active if AutoSPI is enabled."
        n85 = Unbundle By Name(w215) -> ("AutoSPI Active?"=w214:bool)
        n86 = case shown="True" w214 {
          tunnel: [w220 w238] -> w218
          tunnel: w217 -> [w219 w221]
          tunnel: [w219 w228] -> w216
          tunnel: w215 -> [w220 w225]
          tunnel: w215 -> [_ w222]
          frame False {
          }
          frame True {
            n87 = Unbundle By Name(w222) -> ("Reset"=w236:bool, "Data"=w231:dbl[], "Bytes Per Sample"=w235:u32)
            n88 = Unbundle By Name(w222) -> ("TimeStampPrev"=w224:u32)
            n89 = call <vilib>:"FPGA_SPI_ReadAuto.vi"("error in (no error)"=w221, "Bytes per Sample"=w235, "Samples to Read"=u32 0) -> ("error out"=w229:errorcluster, "Timestamps"=w232:u32[], "Data"=w233:u8[][])  [unwired: 6 in]
            n90 = for {
              tunnel: w233 -> [w240] mode=indexing
              tunnel: w232 -> [w243] mode=indexing
              shift-right: [w246] -> w230
              shift-left: w231 -> [w245]
              tunnel: w229 -> [w242]
              tunnel: [w242] -> w228
              shift-right: [w243] -> w223
              shift-left: w224 -> [w244]
              n91 = Subtract(x=w243, y=w244) -> (x-y=w239:u32)
              n92 = call "ADIS16470 Scale Data.vi"("TimeStamp"=w239, "Data In"=w240) -> ("Scaled Data Out"=w241:dbl[])  [unwired: 3 in]
              n93 = Add(x=w245, y=w241) -> (x+y=w246:dbl[])
            }
            n94 = Select(t=dbl[] [0.0, 0.0, 0.0, 0.0, 0.0, 0.0, 0.0, 0.0] ("Angle and Vel"), s=w236, f=w230) -> (s? t:f=w226:dbl[])
            n95 = Bundle By Name(cluster=w225, "Reset"=FALSE ("First Run"), "Data"=w226, "TimeStampPrev"=w223) -> (w238:T16)
          }
        }
      }
      frame "Process" {
        # "#NOTE Move wait here to get data to users faster"
        n96 = Unbundle By Name(w263) -> ("ADIS16470DevRef.Sychronous Process VI"=w258:T8, "ADIS16470DevRef.Data FIFO"=w262:refnum<k33>, "Data"=w257:dbl[])
        n97 = Index Array(array=w257) -> (element #1=w256:dbl, element #2=w255:dbl, element #3=w254:dbl)  [unwired: 3 in]
        n98 = Bundle By Name(cluster="element", "XAngle"=w256, "YAngle"=w255, "ZAngle"=w254) -> (w252:T2)
        n99 = RT FIFO Write(0:w262, 1:w252) -> ()  [unwired: 3 in, 4 out]
        n100 = Not A Number/Path/Refnum?(number/path/refnum=w258) -> (NaN/Path/Refnum?=w259:bool)
        n101 = case shown="False" w259 {
          tunnel: w261 -> [w264 w269]
          tunnel: w252 -> [_ _]
          tunnel: [w268 w269] -> w260
          tunnel: w258 -> [w267 _]
          frame False {
            n102 = call-by-ref "?"(reference=w267, error in=w264, 8:"error in (no error)"=w264) -> (error out=w265:errorcluster, 0:"error out"=w266:errorcluster)  [unwired: 10 in, 1 out]
            n103 = Merge Errors(w265, w266) -> (w268:errorcluster)
          }
          frame True {
          }
        }
        n104 = Wait (ms)(milliseconds to wait=u32 10) -> ()  [unwired: 1 out]
        n105 = Select(t=ADIS16470_Loop_State."Run Cmds Alt", s=w247, f=ADIS16470_Loop_State."Run Cmds" ("ADIS16470 Loop State")) -> (s? t:f=w250:T15)
      }
      frame "Run Cmds" {
        # "#NOTE Should each of these always execute RUN next?\nIf exiting autoSPI to do recalibrate should RUN be skipped\nfor processing another command??"
        n106 = Unbundle By Name(w272) -> ("ADIS16470DevRef.Cmd FIFO"=w282:refnum<k33>)
        n107 = Unbundle By Name(w272) -> ("SPIDevRef"=w271:T17, "ADIS16470DevRef.Status FIFO"=w277:refnum<k33>, "ADIS16470DevRef.Calibration Complete"=w278:refnum<notifier>)
        n108 = RT FIFO Read(0:w282, 1:T20 {"Command"=enum."None", "Data"=0} ("element")) -> (8:w276:refnum<k33>, 9:w275:T20)  [unwired: 2 in, 3 out]
        n109 = Unbundle By Name(w275) -> ("Command"=w274:T24, "Data"=w273:u32)
        n110 = case shown="\"Recal Complete\"" w274 {
          tunnel: w272 -> [w284 w289 w297 w302 w316 w325 w370]
          tunnel: w281 -> [w285 w288 w292 w300 w321 w348 w380]
          tunnel: [w285 w288 w291 w299 w321 w331 w368] -> w280
          tunnel: [w284 w287 w297 w303 w315 w324 w370] -> w279
          tunnel: w278 -> [_ _ _ _ w320 _ _]
          tunnel: w277 -> [_ _ _ w307 w318 _ _]
          tunnel: w276 -> [_ _ _ w305 _ w346 w382]
          tunnel: w273 -> [_ _ w293 _ _ _ _]
          tunnel: w272 -> [_ _ _ _ _ w345 w373]
          tunnel: w271 -> [_ _ w290 w298 _ w322 _]
          frame "None", Default {
          }
          frame "Reset" {
            n111 = Bundle By Name(cluster=w289, "Reset"=TRUE ("First Run")) -> (w287:T16)
          }
          frame "Set Calibration Period" {
            w295 = T14 102 items=["Reserved1"=0, "DIAG_STAT"=2, "X_GYRO_LOW"=4, "X_GYRO_OUT"=6, "Y_GYRO_LOW"=8, "Y_GYRO_OUT"=10, "Z_GYRO_LOW"=12, "Z_GYRO_OUT"=14, "X_ACCL_LOW"=16, "X_ACCL_OUT"=18, "Y_ACCL_LOW"=20, "Y_ACCL_OUT"=22, "Z_ACCL_LOW"=24, "Z_ACCL_OUT"=26, "TEMP_OUT"=28, "TIME_STAMP"=30, "Reseved2"=32, "DATA_CNTR"=34, "X_DELTANG_LOW"=36, "X_DELTANG_OUT"=38, "Y_DELTANG_LOW"=40, "Y_DELTANG_OUT"=42, "Z_DELTANG_LOW"=44, "Z_DELTANG_OUT"=46, "X_DELTVEL_LOW"=48, "X_DELTVEL_OUT"=50, "Y_DELTVEL_LOW"=52, "Y_DELTVEL_OUT"=54, "Z_DELTVEL_LOW"=56, "Z_DELTVEL_OUT"=58, "Reserved3"=60, "Reserved4"=62, "XG_BIAS_LOW"=64, "XG_BIAS_HIGH"=66, "YG_BIAS_LOW"=68, "YG_BIAS_OUT"=70, "ZG_BIAS_LOW"=72, "ZG_BIAS_OUT"=74, "XA_BIAS_LOW"=76, "XA_BIAS_HIGH"=78, "YA_BIAS_LOW"=80, "YA_BIAS_OUT"=82, "ZA_BIAS_LOW"=84, "ZA_BIAS_OUT"=86, "Reserved5"=88, "Reserved6"=90, "FILT_CTRL"=92, "Reserved5"=94, "MSC_CTRL"=96, "UP_SCALE"=98, "DEC_RATE"=100, "NULL_CNFG"=102, "GLOB_CMD"=104, "Reserved6"=106, "FIRM_REV"=108, "FIRM_DM"=110, "FIRM_Y"=112, "PROD_ID"=114, "SERIAL_NUM"=116, "USER_SCR1"=118, "USER_SCR2"=120, "USER_SCR3"=122, "FLSHCNT_LOW"=124, "FLSHCNT_HIGH"=126] ("Register")
            w296 = 1792  # Data
            n112 = Or(x=w293, y=w296) -> (x .or. y?=w294:u32)
            n113 = call "ADIS16470 Write Register.vi"("error in (no error)"=w292, "Data"=w294, "Register"=w295, "SPIDevRef in"=w290) -> ("error out"=w291:errorcluster)  [unwired: 6 in, 1 out]
          }
          frame "Recalibrate" {
            w308 = T14 104 items=["Reserved1"=0, "DIAG_STAT"=2, "X_GYRO_LOW"=4, "X_GYRO_OUT"=6, "Y_GYRO_LOW"=8, "Y_GYRO_OUT"=10, "Z_GYRO_LOW"=12, "Z_GYRO_OUT"=14, "X_ACCL_LOW"=16, "X_ACCL_OUT"=18, "Y_ACCL_LOW"=20, "Y_ACCL_OUT"=22, "Z_ACCL_LOW"=24, "Z_ACCL_OUT"=26, "TEMP_OUT"=28, "TIME_STAMP"=30, "Reseved2"=32, "DATA_CNTR"=34, "X_DELTANG_LOW"=36, "X_DELTANG_OUT"=38, "Y_DELTANG_LOW"=40, "Y_DELTANG_OUT"=42, "Z_DELTANG_LOW"=44, "Z_DELTANG_OUT"=46, "X_DELTVEL_LOW"=48, "X_DELTVEL_OUT"=50, "Y_DELTVEL_LOW"=52, "Y_DELTVEL_OUT"=54, "Z_DELTVEL_LOW"=56, "Z_DELTVEL_OUT"=58, "Reserved3"=60, "Reserved4"=62, "XG_BIAS_LOW"=64, "XG_BIAS_HIGH"=66, "YG_BIAS_LOW"=68, "YG_BIAS_OUT"=70, "ZG_BIAS_LOW"=72, "ZG_BIAS_OUT"=74, "XA_BIAS_LOW"=76, "XA_BIAS_HIGH"=78, "YA_BIAS_LOW"=80, "YA_BIAS_OUT"=82, "ZA_BIAS_LOW"=84, "ZA_BIAS_OUT"=86, "Reserved5"=88, "Reserved6"=90, "FILT_CTRL"=92, "Reserved5"=94, "MSC_CTRL"=96, "UP_SCALE"=98, "DEC_RATE"=100, "NULL_CNFG"=102, "GLOB_CMD"=104, "Reserved6"=106, "FIRM_REV"=108, "FIRM_DM"=110, "FIRM_Y"=112, "PROD_ID"=114, "SERIAL_NUM"=116, "USER_SCR1"=118, "USER_SCR2"=120, "USER_SCR3"=122, "FLSHCNT_LOW"=124, "FLSHCNT_HIGH"=126] ("Register")
            w311 = u16 1  # Data
            # "Write Calibration"
            # "GLOB_CMD Timing"
            n114 = RT FIFO Write(0:w307, 1:T19 {"Calibrated?"=FALSE, "IMU Detected?"=TRUE} ("element")) -> ()  [unwired: 3 in, 4 out]
            n115 = RT FIFO Write(0:w305, 1:T20 {"Command"=enum."Start Auto SPI", "Data"=0} ("element")) -> ()  [unwired: 3 in, 4 out]
            n116 = call "ADIS16470 Write Register.vi"("error in (no error)"=w300, "Data"=w311, "Register"=w308, "SPIDevRef in"=w298) -> ("error out"=w310:errorcluster, "SPIDevRef out"=w309:T17)  [unwired: 6 in]
            n117 = flat-sequence {
              tunnel: w310 -> [w313]
              tunnel: [w313] -> w299
              tunnel: w309 -> [_]
              frame #0 {
                n118 = Wait (ms)(milliseconds to wait=u32 50) -> ()  [unwired: 1 out]
              }
            }
            n119 = Bundle By Name(cluster=w302, "Reset"=TRUE) -> (w303:T16)
          }
          frame "Recal Complete" {
            n120 = Send Notification(notification="", notifier=w320) -> ()  [unwired: 1 in, 2 out]
            n121 = RT FIFO Write(0:w318, 1:T19 {"Calibrated?"=TRUE, "IMU Detected?"=TRUE} ("element")) -> ()  [unwired: 3 in, 4 out]
            n122 = Bundle By Name(cluster=w316, "AutoSPI Active?"=TRUE) -> (w315:T16)
          }
          frame "Exit Auto SPI" {
            w341 = T14 114 items=["Reserved1"=0, "DIAG_STAT"=2, "X_GYRO_LOW"=4, "X_GYRO_OUT"=6, "Y_GYRO_LOW"=8, "Y_GYRO_OUT"=10, "Z_GYRO_LOW"=12, "Z_GYRO_OUT"=14, "X_ACCL_LOW"=16, "X_ACCL_OUT"=18, "Y_ACCL_LOW"=20, "Y_ACCL_OUT"=22, "Z_ACCL_LOW"=24, "Z_ACCL_OUT"=26, "TEMP_OUT"=28, "TIME_STAMP"=30, "Reseved2"=32, "DATA_CNTR"=34, "X_DELTANG_LOW"=36, "X_DELTANG_OUT"=38, "Y_DELTANG_LOW"=40, "Y_DELTANG_OUT"=42, "Z_DELTANG_LOW"=44, "Z_DELTANG_OUT"=46, "X_DELTVEL_LOW"=48, "X_DELTVEL_OUT"=50, "Y_DELTVEL_LOW"=52, "Y_DELTVEL_OUT"=54, "Z_DELTVEL_LOW"=56, "Z_DELTVEL_OUT"=58, "Reserved3"=60, "Reserved4"=62, "XG_BIAS_LOW"=64, "XG_BIAS_HIGH"=66, "YG_BIAS_LOW"=68, "YG_BIAS_OUT"=70, "ZG_BIAS_LOW"=72, "ZG_BIAS_OUT"=74, "XA_BIAS_LOW"=76, "XA_BIAS_HIGH"=78, "YA_BIAS_LOW"=80, "YA_BIAS_OUT"=82, "ZA_BIAS_LOW"=84, "ZA_BIAS_OUT"=86, "Reserved5"=88, "Reserved6"=90, "FILT_CTRL"=92, "Reserved5"=94, "MSC_CTRL"=96, "UP_SCALE"=98, "DEC_RATE"=100, "NULL_CNFG"=102, "GLOB_CMD"=104, "Reserved6"=106, "FIRM_REV"=108, "FIRM_DM"=110, "FIRM_Y"=112, "PROD_ID"=114, "SERIAL_NUM"=116, "USER_SCR1"=118, "USER_SCR2"=120, "USER_SCR3"=122, "FLSHCNT_LOW"=124, "FLSHCNT_HIGH"=126] ("ADIS16448 Register")
            n123 = Unbundle By Name(w345) -> ("ADIS16470DevRef.Hardware Config.IMU SPI Bus"=w344:T7, "ADIS16470DevRef.Hardware Config.SPI Clock Rate (Hz)"=w343:dbl, "ADIS16470DevRef.Hardware Config.IMU SPI Mode (3)"=w342:T5)
            n124 = call <vilib>:"WPI_SPIClose.vi"("error in (no error)"=w348, "SPIDevRef"=w322) -> ("error out"=w327:errorcluster)  [unwired: 9 in]
            n125 = call <vilib>:"WPI_DigitalOutputRefNum Registry Get.vi"("error in (no error)"=w327, "refnum name"="470 Status LED") -> ("error out"=w329:errorcluster, "DigitalOutputDevRef"=w328:T21)  [unwired: 8 in]
            n126 = call <vilib>:"WPI_DigitalOutputSetValue.vi"("error in (no error)"=w329, "Value"=TRUE, "DigitalOutputDevRef"=w328) -> ("error out"=w326:errorcluster)  [unwired: 7 in, 1 out]
            n127 = RT FIFO Write(0:w346, 1:T20 {"Command"=enum."Recalibrate", "Data"=0} ("element")) -> ()  [unwired: 3 in, 4 out]
            n128 = call <vilib>:"WPI_SPIOpen.vi"("error in"=w326, "Mode (3)"=w342, "Clock Rate (Hz)"=w343, "SPI Bus"=w344) -> ("error out"=w340:errorcluster, "SPIDevRef"=w333:T17)  [unwired: 6 in]
            n129 = call "ADIS16470 Read Register.vi"("error in (no error)"=w340, "ADIS16470 Register"=w341, "SPIDevRef in"=w333) -> ("error out"=w334:errorcluster, "Register Value"=w332:u16, "SPIDevRef out"=w335:T17)  [unwired: 6 in]
            n130 = Or(x=u16 16982 ("y"), y=u16 16470) -> (x .or. y?=w337:u16)
            n131 = Equal?(x=w337, y=w332) -> (x = y?=w336:bool)
            n132 = case shown="True" w336 {
              tunnel: w335 -> [_ w362]
              tunnel: w334 -> [w351 w361]
              tunnel: [w350 w360] -> w331
              tunnel: w325 -> [w349 w358]
              tunnel: [w349 w357] -> w324
              frame False {
                n133 = case shown="No Error" w351 {
                  selector: w351 -> [w353 w356]
                  tunnel: [w352 w356] -> w350
                  frame No Error {
                    n134 = call <vilib>:"Error Cluster From Error Code.vi"("error in (no error)"=w353, "error message (\"\")"="SPI port did not reset properly" ("error message (\"\")"), "error code (0)"=-8106) -> ("error out"=w352:errorcluster)  [unwired: 6 in]
                  }
                  frame Error {
                  }
                }
              }
              frame True {
                n135 = call <vilib>:"WPI_SPIRefNum Registry Set.vi"("error in (no error)"=w361, "refnum name"="AutoSPI", "SPIDevRef"=w362) -> ("error out"=w360:errorcluster, "SPIDevRef"=w363:T17)  [unwired: 7 in]
                n136 = Bundle By Name(cluster=w358, "SPIDevRef"=w363, "AutoSPI Active?"=FALSE) -> (w357:T16)
              }
            }
          }
          frame "Start Auto SPI" {
            n137 = Unbundle By Name(w373) -> ("Digital Source"=w372:T9, "SPIDevRef.SPI Bus"=w367:T7, "ADIS16470DevRef.Hardware Config.Stall Config"=w366:T23, "Data Packet"=w365:T14[])
            n138 = RT FIFO Write(0:w382, 1:T20 {"Command"=enum."Recal Complete", "Data"=0} ("element")) -> ()  [unwired: 3 in, 4 out]
            n139 = call <vilib>:"FPGA_SPI_ConfigureAuto.vi"("SPI Auto Zero Byte Count"=u8 0, "error in"=w380, "SPI Auto TX Byte Array"=w365, "Stall Config"=w366, "SPI Bus"=w367) -> ("error out"=w371:errorcluster)  [unwired: 6 in]
            n140 = call <vilib>:"FPGA_SPI_StartAuto_External.vi"("error in (no error)"=w371, "Falling Edge"=FALSE, "Rising Edge"=TRUE, "Source"=w372) -> ("error out"=w377:errorcluster)  [unwired: 7 in]
            n141 = call <vilib>:"WPI_DigitalOutputRefNum Registry Get.vi"("error in (no error)"=w377, "refnum name"="470 Status LED") -> ("error out"=w376:errorcluster, "DigitalOutputDevRef"=w375:T21)  [unwired: 8 in]
            n142 = call <vilib>:"WPI_DigitalOutputSetValue.vi"("error in (no error)"=w376, "Value"=FALSE, "DigitalOutputDevRef"=w375) -> ("error out"=w368:errorcluster)  [unwired: 7 in, 1 out]
          }
        }
      }
      frame "** Register Read Operation **" {
        # "should never get here."
      }
      frame "Run Alt" {
        # "#NOTE JAS Move wait to process"
        # "Main data capture and accumulation loop. Only active if AutoSPI is enabled."
        n143 = Unbundle By Name(w406) -> ("Reset"=w402:bool, "Data"=w401:dbl[], "SPIDevRef"=w395:T17, "Bytes Per Sample"=w391:u32)
        n144 = call "ADIS16470 Read Multiple Registers.vi"("error in (no error)"=w408, "Registers"=w404, "SPIDevRefIn"=w395) -> ("error out"=w407:errorcluster, "Values"=w394:u16[])  [unwired: 6 in, 1 out]
        n145 = Initialize Array(u8 0 ("element"), w391) -> (w393:u8[])
        n146 = for {
          shift-right: [w412] -> w389
          shift-left: w393 -> [w416]
          tunnel: w394 -> [w411] mode=indexing
          tunnel: w390 -> [w410] mode=indexing
          # "hi\nlow"
          n147 = Increment(x=w410) -> (x+1=w415:i32)
          n148 = Split Number(x=w411) -> (hi(x)=w414:u8, lo(x)=w413:u8)
          n149 = Replace Array Subset(array=w416, new element #1=w414, index #1=w410, new element #2=w413, index #2=w415) -> (w412:u8[])
        }
        n150 = call <vilib>:"Util_GetTime.vi"() -> ("FPGA_Time_Seconds"=w388:dbl)  [unwired: 10 in, 1 out]
        n151 = feedback-in #1(w388) -> ()
        n152 = feedback #1(w388) -> (w387:dbl)
        n153 = Subtract(x=w388, y=w387) -> (x-y=w396:dbl)
        n154 = call "ADIS16470 Scale Data Register.vi"("TimeStamp"=w396, "Data In"=w389) -> ("Scaled Data Out"=w397:dbl[])  [unwired: 3 in]
        n155 = Add(x=w401, y=w397) -> (x+y=w400:dbl[])
        n156 = Select(t=dbl[] [0.0, 0.0, 0.0, 0.0, 0.0, 0.0, 0.0, 0.0] ("Angle and Vel"), s=w402, f=w400) -> (s? t:f=w398:dbl[])
        n157 = Bundle By Name(cluster=w406, "Reset"=FALSE ("First Run"), "Data"=w398) -> (w409:T16)
      }
      frame "Run Cmds Alt" {
        n158 = Unbundle By Name(w419) -> ("ADIS16470DevRef.Cmd FIFO"=w429:refnum<k33>)
        n159 = Unbundle By Name(w419) -> ("SPIDevRef"=w418:T17, "ADIS16470DevRef.Status FIFO"=w424:refnum<k33>, "ADIS16470DevRef.Calibration Complete"=w425:refnum<notifier>)
        n160 = RT FIFO Read(0:w429, 1:T20 {"Command"=enum."None", "Data"=0} ("element")) -> (8:w423:refnum<k33>, 9:w422:T20)  [unwired: 2 in, 3 out]
        n161 = Unbundle By Name(w422) -> ("Command"=w421:T24, "Data"=w420:u32)
        n162 = case shown="\"Exit Auto SPI\"" w421 {
          tunnel: w419 -> [w431 w436 w444 w449 w463 w469 w474]
          tunnel: w428 -> [w432 w435 w439 w447 w468 w470 w473]
          tunnel: [w432 w435 w438 w446 w468 w470 w473] -> w427
          tunnel: [w431 w434 w444 w450 w462 w469 w474] -> w426
          tunnel: w425 -> [_ _ _ _ w467 _ _]
          tunnel: w424 -> [_ _ _ w454 w465 _ _]
          tunnel: w423 -> [_ _ _ w452 _ w471 w475]
          tunnel: w420 -> [_ _ w440 _ _ _ _]
          tunnel: w419 -> [_ _ _ _ _ _ _]
          tunnel: w418 -> [_ _ w437 w445 _ _ _]
          frame "None", Default {
          }
          frame "Reset" {
            n163 = Bundle By Name(cluster=w436, "Reset"=TRUE ("First Run")) -> (w434:T16)
          }
          frame "Set Calibration Period" {
            w442 = T14 102 items=["Reserved1"=0, "DIAG_STAT"=2, "X_GYRO_LOW"=4, "X_GYRO_OUT"=6, "Y_GYRO_LOW"=8, "Y_GYRO_OUT"=10, "Z_GYRO_LOW"=12, "Z_GYRO_OUT"=14, "X_ACCL_LOW"=16, "X_ACCL_OUT"=18, "Y_ACCL_LOW"=20, "Y_ACCL_OUT"=22, "Z_ACCL_LOW"=24, "Z_ACCL_OUT"=26, "TEMP_OUT"=28, "TIME_STAMP"=30, "Reseved2"=32, "DATA_CNTR"=34, "X_DELTANG_LOW"=36, "X_DELTANG_OUT"=38, "Y_DELTANG_LOW"=40, "Y_DELTANG_OUT"=42, "Z_DELTANG_LOW"=44, "Z_DELTANG_OUT"=46, "X_DELTVEL_LOW"=48, "X_DELTVEL_OUT"=50, "Y_DELTVEL_LOW"=52, "Y_DELTVEL_OUT"=54, "Z_DELTVEL_LOW"=56, "Z_DELTVEL_OUT"=58, "Reserved3"=60, "Reserved4"=62, "XG_BIAS_LOW"=64, "XG_BIAS_HIGH"=66, "YG_BIAS_LOW"=68, "YG_BIAS_OUT"=70, "ZG_BIAS_LOW"=72, "ZG_BIAS_OUT"=74, "XA_BIAS_LOW"=76, "XA_BIAS_HIGH"=78, "YA_BIAS_LOW"=80, "YA_BIAS_OUT"=82, "ZA_BIAS_LOW"=84, "ZA_BIAS_OUT"=86, "Reserved5"=88, "Reserved6"=90, "FILT_CTRL"=92, "Reserved5"=94, "MSC_CTRL"=96, "UP_SCALE"=98, "DEC_RATE"=100, "NULL_CNFG"=102, "GLOB_CMD"=104, "Reserved6"=106, "FIRM_REV"=108, "FIRM_DM"=110, "FIRM_Y"=112, "PROD_ID"=114, "SERIAL_NUM"=116, "USER_SCR1"=118, "USER_SCR2"=120, "USER_SCR3"=122, "FLSHCNT_LOW"=124, "FLSHCNT_HIGH"=126] ("Register")
            w443 = 1792  # Data
            n164 = Or(x=w440, y=w443) -> (x .or. y?=w441:u32)
            n165 = call "ADIS16470 Write Register.vi"("error in (no error)"=w439, "Data"=w441, "Register"=w442, "SPIDevRef in"=w437) -> ("error out"=w438:errorcluster)  [unwired: 6 in, 1 out]
          }
          frame "Recalibrate" {
            w455 = T14 104 items=["Reserved1"=0, "DIAG_STAT"=2, "X_GYRO_LOW"=4, "X_GYRO_OUT"=6, "Y_GYRO_LOW"=8, "Y_GYRO_OUT"=10, "Z_GYRO_LOW"=12, "Z_GYRO_OUT"=14, "X_ACCL_LOW"=16, "X_ACCL_OUT"=18, "Y_ACCL_LOW"=20, "Y_ACCL_OUT"=22, "Z_ACCL_LOW"=24, "Z_ACCL_OUT"=26, "TEMP_OUT"=28, "TIME_STAMP"=30, "Reseved2"=32, "DATA_CNTR"=34, "X_DELTANG_LOW"=36, "X_DELTANG_OUT"=38, "Y_DELTANG_LOW"=40, "Y_DELTANG_OUT"=42, "Z_DELTANG_LOW"=44, "Z_DELTANG_OUT"=46, "X_DELTVEL_LOW"=48, "X_DELTVEL_OUT"=50, "Y_DELTVEL_LOW"=52, "Y_DELTVEL_OUT"=54, "Z_DELTVEL_LOW"=56, "Z_DELTVEL_OUT"=58, "Reserved3"=60, "Reserved4"=62, "XG_BIAS_LOW"=64, "XG_BIAS_HIGH"=66, "YG_BIAS_LOW"=68, "YG_BIAS_OUT"=70, "ZG_BIAS_LOW"=72, "ZG_BIAS_OUT"=74, "XA_BIAS_LOW"=76, "XA_BIAS_HIGH"=78, "YA_BIAS_LOW"=80, "YA_BIAS_OUT"=82, "ZA_BIAS_LOW"=84, "ZA_BIAS_OUT"=86, "Reserved5"=88, "Reserved6"=90, "FILT_CTRL"=92, "Reserved5"=94, "MSC_CTRL"=96, "UP_SCALE"=98, "DEC_RATE"=100, "NULL_CNFG"=102, "GLOB_CMD"=104, "Reserved6"=106, "FIRM_REV"=108, "FIRM_DM"=110, "FIRM_Y"=112, "PROD_ID"=114, "SERIAL_NUM"=116, "USER_SCR1"=118, "USER_SCR2"=120, "USER_SCR3"=122, "FLSHCNT_LOW"=124, "FLSHCNT_HIGH"=126] ("Register")
            w458 = u16 1  # Data
            # "Write Calibration"
            # "GLOB_CMD Timing"
            n166 = RT FIFO Write(0:w454, 1:T19 {"Calibrated?"=FALSE, "IMU Detected?"=TRUE} ("element")) -> ()  [unwired: 3 in, 4 out]
            n167 = RT FIFO Write(0:w452, 1:T20 {"Command"=enum."Start Auto SPI", "Data"=0} ("element")) -> ()  [unwired: 3 in, 4 out]
            n168 = call "ADIS16470 Write Register.vi"("error in (no error)"=w447, "Data"=w458, "Register"=w455, "SPIDevRef in"=w445) -> ("error out"=w457:errorcluster, "SPIDevRef out"=w456:T17)  [unwired: 6 in]
            n169 = flat-sequence {
              tunnel: w457 -> [w460]
              tunnel: [w460] -> w446
              tunnel: w456 -> [_]
              frame #0 {
                n170 = Wait (ms)(milliseconds to wait=u32 50) -> ()  [unwired: 1 out]
              }
            }
            n171 = Bundle By Name(cluster=w449, "Reset"=TRUE) -> (w450:T16)
          }
          frame "Recal Complete" {
            n172 = Send Notification(notification="", notifier=w467) -> ()  [unwired: 1 in, 2 out]
            n173 = RT FIFO Write(0:w465, 1:T19 {"Calibrated?"=TRUE, "IMU Detected?"=TRUE} ("element")) -> ()  [unwired: 3 in, 4 out]
            n174 = Bundle By Name(cluster=w463, "AutoSPI Active?"=TRUE) -> (w462:T16)
          }
          frame "Exit Auto SPI" {
            # "#NOTE Reg mode doesnt use Auto SPI"
            n175 = RT FIFO Write(0:w471, 1:T20 {"Command"=enum."Recalibrate", "Data"=0} ("element")) -> ()  [unwired: 3 in, 4 out]
          }
          frame "Start Auto SPI" {
            # "#NOTE Register mode doesn't use Auto SPI.  Do nothing."
            n176 = RT FIFO Write(0:w475, 1:T20 {"Command"=enum."Recal Complete", "Data"=0} ("element")) -> ()  [unwired: 3 in, 4 out]
          }
        }
      }
    }
  }
  n177 = flat-sequence {
    tunnel: w7 -> [_]
    frame #0 {
      n178 = call <vilib>:"WPI_DigitalOutputRefNum Registry Get.vi"("refnum name"="470 Status LED") -> ("error out"=w486:errorcluster, "DigitalOutputDevRef"=w485:T21)  [unwired: 9 in]
      n179 = call <vilib>:"WPI_DigitalOutputClose.vi"("error in (no error)"=w486, "DigitalOutputDevRef"=w485) -> ("error out"=w484:errorcluster)  [unwired: 9 in]
      n180 = call <vilib>:"WPI_DigitalOutputRefNum Registry Get.vi"("error in (no error)"=w484, "refnum name"="470 Reset Pin") -> ("error out"=w482:errorcluster, "DigitalOutputDevRef"=w481:T21)  [unwired: 8 in]
      n181 = call <vilib>:"WPI_DigitalOutputClose.vi"("error in (no error)"=w482, "DigitalOutputDevRef"=w481) -> ("error out"=w480:errorcluster)  [unwired: 9 in]
      n182 = call <vilib>:"WPI_SPIRefNum Registry Get.vi"("error in (no error)"=w480, "refnum name"="AutoSPI") -> ("error out"=w478:errorcluster, "SPIDevRef"=w477:T17)  [unwired: 8 in]
      n183 = call <vilib>:"WPI_SPIClose.vi"("error in (no error)"=w478, "SPIDevRef"=w477) -> ()  [unwired: 9 in, 1 out]
    }
    frame #1 {
      n184 = Stop() -> ()  [unwired: 1 in]
    }
  }
  n185 = flat-sequence {
    tunnel: w7 -> [_]
    frame #0 {
      n186 = call <vilib>:"WPI_UtilitiesFRC SendMessageToConsole.vi"("Message"="ADIS16470 Acquisition loop exiting.") -> ()  [unwired: 14 in, 1 out]
    }
  }
